vi "ORCAFusionfor3D250213.vi"(1 "V Offset":i32=1008 min=0 max=2004 step=4, 2 "Exposure":dbl=0.005 min=6.576470588235294e-05 max=10.000017235294118 step=1e-08, 3 "V Width":i32=300 min=4 max=1296 step=4) -> ()   [LabVIEW 2024]
uses:
  <vilib>/vision/driver/IMAQdx.llb/IMAQdx Acquisition Mode.ctl
  <vilib>/vision/driver/IMAQdx.llb/IMAQdx Buffer Number Mode.ctl
  Global variables/filepath global variable.vi
  Global variables/Global 1.vi
  Global variables/global for picoscope.vi
  <vilib>/Utility/file.llb/Write Delimited Spreadsheet (DBL).vi
  Global variables/Global for awg.vi
  <vilib>/Utility/file.llb/Read Delimited Spreadsheet (DBL).vi
  <vilib>/regexp/Match Regular Expression.xnode
  RIGOL DG4000 Series/RIGOL DG4000 Series.lvlib
  <vilib>/vision/driver/NI_Vision_Acquisition_Software.lvlib
  <resource>/objmgr/imaqdx.rc
panel:
  in  "use most recent 2":bool=TRUE
  in  "folder for imgcalib.txt":path=path "E:/20250409-103904beads-cropbulkcalib"
  in  "copy later":bool
  out "UDP wait":i32=236
  out "result":bool
  in  "force stop":bool
  out "time ofst":dbl=2434.2794585227757
  out "Image":u16[][](graph)
  in  "force 2":bool
  out "rec ready":bool
  in  "force":bool
  in  "master IP":string="192.168.11.3"
  out "Frame Count 2":i32=1726
  out "Frame Index":i32=1725
  out "error out 6":errorcluster
  out "error out 5":errorcluster
  in  "UDP send at monitor":bool
  in  "save BF video":bool
  out "error out 4":errorcluster
  in  "Stop (F)":bool
  out "BF save idx":i32=157
  out "Tot Img Trans":u32=158
  out "Lost Imgs":u32
  in  "error in 2":errorcluster caption="error in"
  out "buffers to read":i32=1
  in  "UDP send vol img":bool=TRUE
  in  "pico send port":u16=61558
  in  "pico receive port":u16=61559
  in  "cam receive port":u16=61551
  in  "cam send port":u16=61550
  in  "img send port":u16=61554
  in  "img receive port":u16=61556
  in  "img process IP":string="169.254.243.60"
  in  "slave IP":string="192.168.11.4"
  in  "ROI ratio [0-1]":dbl=0.40000000000000013 min=0.0 max=12.009207563363388 format="%_3g"
  in  "BF Gain":dbl=1.40920756336339 min=0.0 max=12.009207563363388
  in  "BF Exp Time [us]":dbl=25000.0 min=81.0 max=1000000.0
  in  "picoscope  IP":string="192.168.11.5"
  in  "control picoscope dependent enable":bool
  out "error out 3":errorcluster caption="config save"
  in  "avg":bool
  out "img projection on x":u32[](graph)=[46763, 46566, 47465, 47353, 48054, 49097, 50269, 51790, 53469, 55555, 57972, 59664, 62238, 64752, 68892, 72850, 78469, 84812, 92692, 100027, 109195, 119310, 130289, 140697, 155154, 168575, 186107, 203972, 224307, 243761, 265655, 286409, 306031, 324848, 342017, 357018, 368904, 379402, 387267, 388850, 395332, 391042, 392409, 389360, 387631, 382204, 372553, 361258, 353852, 348315, 349132, 352795, 362226, 378823, 399724, 419608, 438876, 459397, 481066, 502548, 524212, 537389, 551531, 567399, 572506, 575998, 579368, 577266, 572748, 565672, 554518, 543313, 531291, 514913, 503094, 495158, 488186, 477560, 468588, 467112, 458508, 452252, 445557, 436410, 425728, 418022, 407398, 396484, 384057, 369408, 354457, 334333, 315868, 295311, 272375, 251508, 229534, 206536, 185054, 162964, 142104, 125408, 111109, 98736, 88371, 80016, 75159, 71056, 66418, 63549, 62540, 60488, 59786, 59593, 58091, 58342, 57603, 57721, 57813, 58251, 57480, 56985, 56492, 55978, 55882, 55969, 55694, 54777, 55153, 54636, 54366, 54397, 54470, 54398, 53686, 53410, 52884, 53176, 51940, 51877, 51333, 51303, 50817, 50985, 50476, 51047, 50390, 52065, 53983, 54808, 55888, 57189, 58691, 60664, 61183, 62686, 64574, 67089, 71468, 75339, 80938, 88612, 96438, 106174, 117774, 131064, 143808, 162504, 179386, 199476, 221027, 241869, 264955, 289252, 314205, 339403, 360641, 381980, 400735, 413883, 425153, 437700, 437408, 441439, 438854, 433479, 429254, 421027, 412972, 405392, 396731, 386405, 373085, 362958, 361482, 367425, 375402, 388356, 414798, 445670, 475814, 507271, 539682, 567255, 593366, 615447, 634310, 648625, 657756, 659455, 652031, 647118, 635908, 619182, 600572, 575600, 548617, 521219, 489430, 463193, 440358, 414296, 395402, 379226, 362114, 347669, 336524, 321767, 311716, 298256, 290618, 283823, 275246, 264692, 257127, 245035, 235078, 222050, 207522, 192842, 179267, 165496, 150685, 136934, 122505, 112106, 99543, 90769, 83386, 77341, 73424, 69532, 66073, 63964, 61802, 60456, 60172, 58053, 58610, 57914, 57379, 56188, 56799, 56522, 56383, 56136, 56350, 55969, 55894, 55596, 55550, 54966, 54216, 55062, 54752, 54939, 54056, 54219, 54106, 53703, 52919, 52784, 52570, 51188, 51390, 51350, 50853, 51444, 51914, 53286, 54912, 56386, 57845, 59413, 61190, 61964, 62139, 63564, 65517, 66692, 68803, 72468, 75689, 81725, 88028, 96533, 106800, 119624, 134822, 150087, 169629, 188666, 213128, 237819, 265095, 290925, 321363, 352398, 380193, 407341, 429230, 449456, 468115, 478920, 483867, 493482, 494367, 495346, 491733, 479634, 470046, 458955, 444614, 433281, 422348, 410073, 402638, 392584, 389266, 392847, 405373, 422542, 450281, 484856, 524179, 564068, 600997, 635572, 667615, 693349, 710453, 723810, 733326, 733971, 727639, 712926, 695281, 673791, 644151, 611255, 574822, 533808, 489856, 452557, 413089, 378985, 344296, 316157, 288985, 267488, 246789, 230505, 217301, 205969, 197601, 191265, 186443, 180492, 173239, 168631, 161521, 154799, 147874, 139498, 133757, 122991, 117586, 109419, 101760, 94727, 87387, 81708, 76026, 72895, 69737, 65592, 64545, 61762, 61493, 60316, 58335, 58021, 56599, 56717, 56451, 56236, 55904, 55987, 56231, 55048, 55126, 55901, 55591, 54653, 54155, 54580, 54543, 54603, 53867, 54428, 54306, 54044, 53700, 53600, 53539, 53111, 53102, 52748, 52697, 53594, 55555, 57500, 58837, 61645, 64114, 65348, 65886, 67016, 67614, 67654, 69657, 72162, 75056, 78198, 82504, 88800, 96598, 106234, 117020, 131257, 145720, 164156, 182364, 203376, 229013, 257225, 289129, 316516, 351185, 379123, 410151, 437385, 462763, 481027, 499315, 510603, 518971, 520139, 522881, 518519, 516459, 512100, 498143, 485882, 475328, 460116, 450415, 437217, 426723, 420391, 413940, 412723, 419085, 432764, 456433, 485422, 524525, 565162, 610088, 648437, 686398, 718800, 747419, 766010, 777514, 777044, 778427, 763909, 751696, 725442, 695879, 665038, 625739, 585270, 539158, 490792, 441142, 394881, 350379, 311008, 274508, 243018, 216015, 191695, 172900, 158220, 144123, 135334, 129242, 125294, 121970, 118239, 115135, 113271, 108002, 105537, 103368, 98928, 96060, 92167, 88539, 85061, 81133, 76890, 73457, 69890, 68677, 66634, 64257, 61754, 60821, 59558, 58395, 58513, 56328, 56141, 55792, 55574, 55876, 55499, 55004, 55402, 55345, 54894, 54699, 55016, 55041, 54684, 54209, 54577, 54510, 55124, 53770, 53483, 53717, 52644, 53505, 53602, 53088, 52707, 53282, 55024, 57713, 60024, 62878, 66235, 68694, 71215, 72999, 75032, 75858, 78590, 79163, 82438, 84466, 88891, 93706, 101282, 108113, 117174, 128616, 140654, 156941, 173135, 189677, 209640, 233642, 255507, 284400, 314625, 343006, 373109, 405302, 430985, 454705, 479403, 499728, 509992, 522190, 534539, 537888, 540312, 541391, 536423, 533375, 527903, 521478, 511809, 497760, 490753, 481320, 470512, 463190, 455798, 455219, 457499, 463730, 483205, 501868, 534714, 570832, 612318, 653007, 688852, 726270, 755878, 773610, 786847, 793248, 788675, 778998, 762326, 741613, 710124, 680934, 645559, 600535, 559941, 510879, 462833, 411293, 361698, 316739, 276859, 238493, 206282, 177438, 155511, 136038, 121533, 111596, 102609, 98600, 93511, 91228, 90109, 87612, 86054, 84772, 83804, 83650, 81231, 79034, 78308, 76125, 74817, 73368, 71865, 69032, 66726, 66145, 64251, 63185, 62358, 60763, 59310, 58836, 58519, 57076, 57695, 56673, 56647, 56615, 56011, 56065, 55656, 55461, 55662, 55299, 55677, 55908, 55040, 55014, 55895, 55142, 55733, 54291, 54438, 53795, 54601, 55215, 55425, 56957, 59882, 62453, 65632, 68780, 72560, 75412, 79552, 81468, 85046, 88090, 91442, 94344, 97575, 102906, 109576, 119126, 127735, 135862, 149342, 163796, 178621, 197113, 214594, 234706, 252396, 273899, 294607, 316765, 343214, 368638, 393386, 420665, 442983, 464259, 480357, 492508, 500708, 510357, 516660, 524411, 530971, 535190, 536034, 537105, 535876, 532909, 533313, 526314, 519232, 511560, 501525, 495308, 483290, 479364, 479346, 478860, 483300, 492570, 510965, 535881, 562874, 596055, 632312, 662038, 696751, 717383, 742176, 749917, 755987, 746600, 739245, 721556, 703042, 678722, 646019, 613429, 576811, 534667, 494339, 446301, 397380, 352581, 306403, 267865, 228945, 197581, 171555, 148010, 128502, 114118, 103197, 94032, 87802, 82480, 81184, 79017, 77204, 76793, 75420, 74572, 75099, 73593, 73408, 71627, 71309, 70209, 70774, 68776, 67944, 66009, 64393, 64407, 61956, 62331, 60890, 60805, 59475, 58855, 57975, 58083, 56975, 56977, 57278, 56861, 56411, 57107, 56762, 56913, 56257, 55657, 56298, 55799, 55779, 55602, 56401, 54827, 54668, 54422, 55422, 56213, 58272, 60132, 62006, 66355, 68450, 72697, 76562, 79975, 84644, 88439, 94301, 98930, 105254, 111465, 118621, 126709, 135204, 146414, 159222, 173651, 191478, 209063, 229838, 250513, 272267, 291585, 314719, 332340, 352328, 371069, 388356, 408658, 424320, 444853, 460671, 475012, 485228, 494000, 494571, 499023, 498881, 501009, 508428, 513098, 522833, 531481, 533378, 538412, 541736, 542287, 540438, 537292, 533782, 527968, 518489, 511686, 501691, 492153, 489715, 486694, 488329, 492105, 504124, 520584, 539851, 562253, 586323, 615491, 635563, 651874, 659035, 662606, 657157, 647946, 637716, 618358, 600924, 574402, 546181, 516077, 486466, 446289, 412376, 372443, 330677, 292392, 255923, 221850, 192879, 167113, 145811, 127025, 113704, 102444, 94562, 87374, 83407, 77742, 77121, 74132, 73679, 72464, 72005, 71342, 70178, 70459, 69718, 69138, 68748, 68189, 67696, 66799, 65713, 64961, 64463, 63252, 62852, 61849, 60461, 59643, 59776, 58932, 57673, 57651, 57025, 56749, 57710, 58078, 56667, 57160, 56437, 56713, 55969, 55979, 55988, 55737, 55922, 56094, 55446, 56541, 57664, 59499, 61720, 63823, 66018, 69061, 72232, 75368, 79556, 82900, 87771, 93106, 100163, 109727, 119195, 129630, 140138, 153328, 168378, 184368, 202515, 226296, 249446, 274734, 300671, 326457, 349959, 375628, 399007, 417677, 438041, 451834, 467356, 477363, 487782, 497901, 507169, 513957, 516170, 513887, 514861, 513323, 507136, 502739, 499439, 502497, 509217, 519171, 531478, 539064, 548065, 553679, 558886, 560565, 555793, 553298, 548006, 535963, 526058, 509826, 501258, 489039, 480329, 467466, 459027, 455901, 457194, 466412, 472844, 481954, 500378, 515647, 527143, 528788, 532753, 529135, 521695, 511153, 497039, 478216, 461326, 438452, 420035, 397745, 368464, 341391, 311948, 280824, 253865, 222955, 195390, 170664, 149175, 132071, 118878, 108688, 99158, 91978, 87181, 83209, 79800, 76421, 74690, 72193, 71263, 70267, 70410, 69170, 69505, 69184, 69134, 68814, 67928, 67770, 66360, 66150, 66109, 64758, 63735, 63081, 61919, 61853, 61632, 60449, 60652, 60128, 59036, 59188, 59063, 58580, 57639, 58652, 58142, 58260, 58426, 58344, 57729, 57843, 57657, 58503, 60967, 62530, 64189, 67978, 69308, 72699, 75598, 76963, 78740, 82423, 86195, 90634, 96316, 104436, 113212, 123960, 135348, 151749, 167657, 187248, 208644, 234661, 261361, 289449, 318033, 347216, 382491, 411942, 443503, 470688, 494191, 513211, 532495, 546968, 559280, 563098, 568707, 574630, 576306, 573994, 574301, 572743, 565857, 556853, 550941, 541122, 530722, 527826, 530160, 537484, 545186, 560363, 573150, 583316, 583372, 584437, 577068, 574591, 566652, 556635, 544800, 530273, 510395, 490442, 472939, 452229, 428681, 407695, 388867, 377702, 370827, 370301, 368389, 371544, 379539, 384309, 387899, 387049, 383115, 373877, 365172, 358048, 345655, 332013, 320266, 301273, 287529, 269564, 252052, 234242, 214021, 193605, 174578, 156405, 139534, 124363, 113613, 106526, 99431, 93531, 88245, 84911, 81424, 78650, 76329, 74234, 72670, 71463, 69882, 70270, 70029, 69343, 68388, 68592, 68126, 68251, 67684, 67107, 66204, 66381, 65869, 65350, 64341, 63657, 62936, 63157, 62354, 62490, 62383, 61429, 61896, 60989, 60215, 60454, 59986, 59353, 60091, 60083, 60272, 61016, 61732, 63650, 66878, 69853, 72409, 76090, 77719, 81626, 83862, 84953, 88525, 91994, 95122, 100678, 106585, 115016, 123268, 134460, 148618, 166605, 184944, 207904, 229903, 260888, 290300, 322193, 358613, 392442, 424837, 465456, 501501, 532401, 561444, 584650, 607106, 623032, 635080, 645734, 653773, 656815, 658544, 656549, 654539, 647014, 646190, 638408, 627915, 619526, 606518, 599238, 589066, 588115, 587987, 596125, 605755, 616686, 623131, 626647, 621152, 609225, 597147, 582436, 566852, 555739, 537492, 514810, 491461, 466012, 439105, 410246, 379739, 348501, 319113, 299635, 283029, 271006, 259836, 257610, 255632, 255968, 256242, 254458, 250537, 245450, 240074, 234972, 227618, 218501, 211862, 202945, 193330, 183380, 173531, 162316, 151819, 141017, 130507, 119635, 110267, 103633, 97552, 92520, 88504, 84892, 82268, 79516, 78045, 75838, 74257, 73572, 71734, 70639, 70069, 70069, 68607, 68328, 68748, 69112, 67981, 67374, 67373, 66304, 66789, 65901, 66062, 64961, 63977, 65245, 64377, 63630, 63604, 63967, 62407, 63214, 62344, 61961, 61774, 61036, 62023, 62930, 65684, 66942, 69995, 76001, 78880, 83373, 86841, 89315, 93801, 94836, 97208, 101451, 106133, 111049, 118204, 124706, 134766, 147204, 161353, 175813, 195481, 216380, 238811, 261184, 292301, 320473, 353593, 390048, 424548, 461921, 498089, 530867, 564423, 595816, 626983, 652126, 671002, 688270, 701533, 713810, 722754, 726314, 729340, 732940, 733028, 731046, 726045, 715923, 704688, 696391, 687102, 683341, 670739, 663697, 661041, 660387, 662810, 669403, 670798, 664673, 656682, 637876, 617533, 589418, 567700, 551910, 532396, 509588, 482087, 454509, 425145, 391865, 358574, 321135, 285411, 254640, 230948, 209641, 195414, 181370, 174427, 167958, 165639, 164684, 160171, 157109, 155233, 153616, 149682, 146704, 142205, 137923, 134356, 129851, 124980, 120013, 114239, 108885, 103690, 99268, 94468, 90762, 86230, 83823, 81021, 78977, 77084, 75557, 74597, 73002, 72729, 71162, 69426, 70028, 69318, 67892, 68868, 67483, 66913, 67287, 67555, 66142, 66315, 67040, 65491, 65669, 65403, 65681, 65224, 65278, 64135, 64150, 63686, 64044, 63637, 63242, 62525, 61698, 62245, 61811, 63049, 64547, 67956, 70609, 75237, 81093, 85648, 93090, 97431, 101731, 106858, 110864, 117654, 122759, 129252, 137895, 145048, 155739, 170843, 185489, 204045, 223243, 243633, 268584, 292435, 317121, 342349, 369902, 399530, 429393, 462446, 496455, 529059, 558314, 587899, 616309, 644410, 666002, 690379, 708113, 731660, 751461, 765659, 782685, 791681, 799765, 805173, 808663, 812066, 807592, 797973, 788513, 775893, 762811, 751623, 741070, 729946, 720074, 717443, 716245, 709738, 702259, 693124, 681834, 662431, 636216, 604702, 574075, 544633, 520712, 497617, 477753, 447300, 416352, 386342, 350714, 316994, 279730, 245240, 215017, 186365, 165427, 149431, 134762, 124069, 117802, 113972, 111451, 108212, 106559, 106003, 104053, 102471, 101832, 99318, 97950, 95984, 94380, 92804, 90925, 87889, 86332, 84699, 81928, 79786, 78244, 76929, 74832, 73871, 71723, 71905, 70749, 69591, 69410, 68104, 67663, 67370, 66572, 65358, 65540, 65770, 65293, 65134, 64461, 64123, 64955, 63954, 63499, 64235, 62877, 63787, 62841, 63494, 62554, 61743, 62057, 61599, 60186, 60950, 60480, 60778, 60657, 62136, 63581, 65769, 69642, 74391, 79857, 85246, 92397, 98998, 107390, 116571, 124545, 131994, 142229, 153291, 163548, 177881, 191992, 207585, 230523, 250293, 273919, 300201, 327896, 357657, 380818, 409210, 434937, 462041, 486284, 512740, 539203, 565531, 588857, 619273, 636650, 657509, 678060, 694261, 715038, 735168, 759656, 775484, 795112, 815744, 839395, 851805, 862003, 870832, 874827, 874824, 869134, 856216, 841567, 821890, 802659, 784915, 768650, 751584, 741555, 731571, 716175, 702050, 688414, 676278, 651137, 627903, 598903, 562873, 530382, 502630, 474887, 452077, 428903, 404965, 378811, 347369, 316651, 285902, 253523, 219876, 191077, 162607, 144229, 127086, 114637, 105398, 97788, 93173, 90056, 87082, 84545, 83619, 83178, 82178, 80760, 79681, 80028, 78757, 77506, 77230, 77014, 76447, 75667, 74473, 74658, 72432, 72148, 71246, 69164, 69417, 68323, 67018, 66728, 65535, 65955, 64540, 64052, 64783, 63809, 63934, 62562, 63125, 63382, 63195, 62089, 62263, 62538, 61898, 62003, 61987, 61715, 60810, 60764, 60289, 59903, 60112, 59165, 58832, 59077, 60239, 60941, 61907, 63578, 65479, 68861, 72721, 78549, 85103, 92676, 100742, 110143, 122825, 137696, 151108, 165849, 181928, 200582, 219123, 240759, 268390, 293942, 322516, 350804, 380186, 415968, 450931, 481132, 512024, 543238, 572639, 595963, 623884, 641402, 667756, 685579, 704673, 719769, 734097, 746735, 756245, 763244, 776213, 785879, 797241, 809994, 830952, 853748, 884065, 898879, 915910, 924958, 929875, 921709, 913768, 902456, 880502, 852432, 821412, 791564, 758247, 733464, 713488, 694840, 679243, 660419, 640481, 619488, 593945, 573547, 543351, 514023, 481765, 451702, 421292, 397609, 376451, 358299, 337797, 314412, 292551, 265775, 242066, 213026, 187817, 163852, 144755, 127914, 114425, 102441, 96208, 90535, 85740, 82498, 79334, 77852, 76006, 75789, 74410, 75163, 73839, 73611, 74269, 72906, 73256, 72890, 71503, 71628, 71277, 71731, 70354, 69625, 69495, 68541, 68131, 66889, 66153, 65214, 64926, 65725, 64831, 64657, 64172, 63755, 63769, 62687, 63541, 63148, 62709, 63217, 62308, 62666, 62670, 62457, 61548, 61571, 61103, 61423, 60534, 59216, 60958, 60785, 61214, 61294, 63337, 63371, 65573, 67443, 69870, 74322, 78052, 84778, 92348, 102626, 112453, 127034, 144489, 166031, 186787, 212098, 238712, 272078, 303589, 336952, 373906, 413511, 449802, 488112, 529905, 572761, 612162, 649537, 684337, 717353, 747525, 780325, 799854, 821516, 842427, 860436, 870764, 876368, 887719, 886533, 886338, 884878, 882939, 878119, 876774, 883135, 887243, 902900, 928355, 950250, 958519, 964094, 967841, 958992, 935840, 917902, 884201, 852477, 806465, 763670, 720665, 681044, 649302, 622608, 599953, 576659, 551065, 526067, 503866, 474630, 449745, 423022, 396999, 370839, 344772, 323190, 302128, 288776, 273658, 258814, 242313, 221669, 204526, 184526, 166382, 151290, 133572, 120289, 109493, 102207, 94856, 91292, 85823, 82481, 81064, 77533, 75875, 75553, 76188, 74126, 74914, 74264, 72800, 72663, 72818, 71612, 73391, 70575, 70713, 70828, 70331, 69837, 69740, 69456, 69369, 69092, 68393, 68244, 65885, 65892, 66170, 65288, 65606, 64420, 64465, 64831, 64243, 63648, 63970, 63360, 63355, 64023, 62883, 62986, 61553, 61221, 61975, 61749, 62484, 62149, 62848, 63036, 63655, 64647, 65540, 66994, 69767, 70452, 73899, 76465, 81806, 86263, 94014, 102961, 115672, 132973, 151256, 174915, 202830, 235405, 270932, 309650, 350970, 402340, 447192, 496732, 541670, 594440, 647322, 690986, 742780, 788664, 829420, 872703, 911922, 945992, 967093, 995894, 1023769, 1044035, 1055736, 1065514, 1067810, 1067918, 1062822, 1056107, 1040368, 1023694, 1004512, 987379, 966399, 958464, 953263, 962909, 973305, 982364, 977187, 967864, 949521, 921940, 892684, 857498, 815282, 763596, 711178, 658337, 607590, 563858, 527965, 500003, 469418, 446141, 419065, 394736, 371463, 347798, 325460, 304621, 286410, 262655, 246715, 231281, 218527, 207951, 196175, 186747, 175289, 162510, 152076, 138768, 127521, 118057, 109188, 102916, 96430, 92342, 88799, 85983, 83518, 81444, 80225, 77409, 76879, 74841, 74356, 74110, 73313, 73319, 72944, 72192, 71987, 71450, 71381, 70868, 69768, 70381, 71173, 69571, 69147, 69153, 68938, 69572, 68696, 66881, 66746, 66779, 67580, 66299, 66488, 65587, 65330, 64789, 65169, 63458, 63127, 64178, 63283, 62548, 61478, 60982, 60950, 60289, 60191, 60949, 60917, 59272, 60064, 59752, 59923, 60254, 60326, 59469, 58715, 59647, 59200, 58036, 58655, 57850, 58271, 57778, 56639, 56055, 56910, 57189, 55912, 56106, 56456, 57093, 56121, 57182, 56239, 55974, 56403, 56361, 55629, 57655, 55400, 56492, 55490, 56104, 56031, 55803, 56218, 55837, 55851]
  out "x-y":i32=1726
  in  "calib":bool
  in  "page":i32
  in  "calib/monitor":bool
  in  "max adjust":dbl=1.0 format="%_2g"
  out "frame's init pos in x":dbl[][](array[numeric])=[[0.0, 0.411157223986379], [140.8042176643056, 140.13608717532782], [280.2664638336562, 281.07735724762904], [420.37970894098385, 420.73947151197183], [560.413006810315, 560.8241640343012], [700.4177520946471, 700.3663574416489], [841.3247590649489, 840.9649964939609], [981.1581888392866, 980.7184790303013], [1120.4405537231426, 1120.9002503416273], [1261.6530733529344, 1261.807257311929], [1401.606423984268, 1401.1952667602816], [1541.9480897715885, 1542.2564576895784], [1682.0013744504195, 1682.700912782896], [1822.705658067228, 1822.9626313322192], [1963.5013099560329, 1963.2471919495415], [2103.2576477508737, 2103.463226362867]]
  out "stop acq":bool
  out "cropcalib ch2 2":dbl[][][](array[numeric])=[[[0.8701974985351326, 12.622808311820734, 0.34821884375588075, -0.03186060376885538], [0.7855164449626466, 12.248049490220744, -1.7933514926448941, -0.02615765607541458], [0.8790915308550922, 12.649388072757741, -1.7193702597053502, -0.03530778831987937], [0.8898204410615707, 12.542700034696967, -1.2340309712985338, -0.0439179338550789], [0.8871233001173581, 12.211143396475, -0.7011267129566395, -0.04065012404196286], [0.8976455855239693, 12.395744078277922, 0.44657632622208226, -0.035478990396647044], [0.6373130758818424, 10.721989467950603, -1.4081455713558404, -0.03444993212203115], [1.0111876965038278, 13.101523969448772, -1.3515523786356038, -0.006328878978959408]], [[0.3516942877029585, 4.921154461560632, -1.4770116333666226, -0.044838979986691584], [0.4586265170701861, 6.290835239491175, -0.5978805404070313, -0.03058477703735147], [0.48928552986839696, 6.246479501151768, -0.8501187541827993, -0.038934055058172115], [0.4704781032593286, 6.085031903419253, -1.2048861241864888, -0.027245570005914273], [0.4829021826517912, 5.720772505452486, -0.31646170698518505, -0.03774629427187434], [0.47432244943347757, 5.744490489126907, 0.3764850609397732, -0.026645671939902214], [0.35735176873885377, 5.155667320753812, -0.6110375964837094, -0.043001090221026814], [0.47169885007454965, 5.719049879710236, -1.214570394374455, -0.0357302420415391]], [[0.42431543103473984, 3.311153310021567, 0.3735087392794577, -0.026078458785932162], [0.4185393774710084, 3.510033946713933, -0.6974826786495143, -0.023717547547826606], [0.40107970241405455, 3.155388779364144, -1.4495184075110343, -0.0272149970173807], [0.4038785451829636, 2.894250692768182, -0.6626971578268964, -0.0325936670560735], [0.43463410117317575, 2.814665468074131, -0.07031969386775042, -0.02770361073912457], [0.45431959379871734, 3.3728460691517603, 0.04004989854315301, -0.02424459784876358], [0.4505805120561091, 3.337447688751297, -1.2625490394650989, -0.026776561893721327], [0.4251020680903856, 3.127743751549204, -0.6429568474166446, -0.02863037070461889]], [[0.3552757546386318, 1.3397492427317914, -0.3215132994421062, -0.025808768004406273], [0.36295246493286104, 2.0006437609736487, -1.3336461209741413, -0.017833549159850304], [0.35855770640942686, 1.8571434623079024, -1.4041148558396288, -0.020755845044606074], [0.4114652020285343, 2.0139473340600365, -0.1937946219538823, -0.02382442826394008], [0.3499301521182933, 1.3389264069092857, -0.21029767748849823, -0.022723031905148013], [0.38059424489364246, 1.5220229333510222, -0.1302571590494475, -0.016263248981750543], [0.4207868671061959, 1.9890909149992932, -0.11465078250135777, -0.019859715040226194], [0.4148040618017305, 1.6458278151709658, -0.41822866513797036, -0.02596361679279958]], [[0.2938047023063933, 0.15848081496267857, 0.21377935785301977, -0.017044009015294515], [0.3578200533394036, 1.440800298674786, -0.25425224089524223, -0.013068948485870282], [0.35091888359219314, 1.346093085991901, 0.03700652414677099, -0.018437088761087322], [0.2615412035983308, 0.2553357946660699, 0.06563804987560529, -0.013729022790036183], [0.27744688808915585, 0.16285376720024541, 0.3969513138143117, -0.024167766761933995], [0.2410317694018692, 0.01719906807802845, 0.31887980936003024, -0.013899480418623898], [0.32670519203836695, 0.7070294256236573, 0.06889024493523768, -0.013849213382843669], [0.26929735820100886, 0.21585137293623718, 0.16764603161195335, -0.017509725152931335]], [[0.23964527052154094, 1.405161828042007, 0.7263938040790185, -0.013558480972783012], [0.23329678829132916, 1.9842641685831914, -0.43751729409466744, -0.009372812399959492], [0.29609136804454006, 2.2197331529484727, -0.3606187984687732, -0.014591349298057148], [0.18364046988106897, 1.0318842702071733, -0.21467102230538426, -0.006974976860324521], [0.237430149883509, 1.1354461619807799, 1.253426813991111, -0.010764567951424628], [0.21428788494745543, 1.2084708667209956, 0.6454519731653344, -0.014856742787382637], [0.19128550557336332, 0.9914202026492045, -0.012966520111932736, -0.01039845002841516], [0.18478085458589122, 0.6855671795600868, -0.05129936188141995, -0.014242565681526993]], [[0.15123693469828958, 1.163110201653609, 0.8745656657567553, -0.006604690732614436], [0.1617626592665295, 1.8451285513720417, -0.22859918528260925, -0.006219911053321165], [0.16565366259007014, 1.6280136877205398, -0.10883101331753334, -0.00964042687757254], [0.10928971110762957, 0.749493310399407, 0.003138228221609993, -0.008573046658971014], [0.02253022817352303, 0.07522041477715277, 0.8174746482416958, -0.007898334309960686], [0.003821773667235064, 0.19087983139285825, 1.2250839805129892, -0.006940107606339307], [0.17999809793891175, 1.4975328046377405, -0.11799490261557272, -0.0031203973369017474], [0.12067298238529153, 0.8183571646791823, 0.21700018598403456, -0.003330307143816533]], [[-0.0005213232213452705, 0.11664433274256322, -0.14703000948528538, 0.0022223370156425545], [-0.004751436308695322, 0.44945437865127735, 0.4407582496415892, 0.0009313311130397984], [-0.04601125513680242, 0.12232865474884935, -0.5555144671157969, -0.008711753743847687], [0.0, 0.0, 0.0, 0.0], [-0.0006907142392795103, 0.0644444433024974, -0.0722068891602118, -0.0030870140283082302], [0.001947573415548731, 0.009430552383996885, 0.376950878453279, 0.004011208280281968], [0.00601799297429685, -0.171200104000229, 0.4028188227208616, -0.0006892635684963884], [-0.0035595026932949752, -0.1639845558444737, 0.20081933970234833, 0.0007759675622934727]], [[-0.0445905899107714, 0.3878308646235794, 0.2999945087607148, 0.0006132606194773083], [-0.0233479900245816, 0.805464715742334, 0.002260800741456181, 0.0007923205997293554], [-0.027075628767392633, 0.21947910469952261, -0.6085871209249598, -0.00044238879126859074], [-0.14801341061316545, -0.9604402676156238, 0.04927742722480564, -0.010081622437758307], [-0.1351946090418747, -1.4037614517100776, 0.19096669008196027, -0.0005919410201843423], [-0.025443865945330033, 0.16995044160417527, -0.1562744263326309, -0.00198507171588911], [-0.017148669006657007, 0.20096477942386526, -0.0948436802257652, -0.0037168132796431656], [-0.045635057561963205, -0.07042763819321216, 0.178354420444418, -0.001384743167300897]], [[-0.14847892629844361, -2.1190919588657353, -0.39668969526474496, -0.003525009441780651], [-0.15170487526883455, -1.517780253977753, 0.40100295859357254, -0.003671659512345847], [-0.15582312230276163, -1.749691739278918, 0.4041461560506011, -0.006519857435921785], [-0.1490680046293541, -2.141748665352092, 0.4764301961883949, -0.0037233647798519207], [-0.19546209831376074, -3.094433551917896, 0.10995617619126552, -0.0013108345240767923], [-0.1663997352333837, -2.5234347104959314, 0.016952984209117655, -0.001558016324829012], [-0.16864610100772026, -2.2519891134627716, 0.009421852652772325, -0.0015948467476679916], [-0.17038719997008178, -2.6042474433647995, 0.09965476021822894, -0.0009880362442417799]], [[-0.1917409778980073, -3.892103482576627, 0.011307393107903144, -0.000973113351354111], [-0.23155366010446854, -3.73698000173536, -0.32159229488976254, 0.0043611241773148105], [-0.2149861492875637, -3.826512088064914, 0.35988121969000053, -0.003276087734406148], [-0.1850914206691932, -3.9073215173591516, -0.2976902305965188, 0.0018181088617474789], [-0.2166956185114457, -4.759035950022652, -0.39731132566536975, -0.0018975172421048176], [-0.18453416290159624, -4.081079332925176, 0.06634914312032889, 0.007699054345041634], [-0.18380968001623293, -3.94398458212836, 0.05540268327058757, 0.0077636042799711326], [-0.17894442370330435, -4.023445572474, 0.174749370962602, 0.005127314289389062]], [[-0.2071791595959074, -5.602941921550978, 0.5697348661401064, -0.004793728154630928], [-0.293851025233213, -6.076200837157158, 0.36633789088880986, -0.014666619442646871], [-0.3125311419595355, -6.474337848680638, -0.46570696369851816, -0.012047430951543585], [-0.2759968219061918, -6.572782260152643, 0.26886806477602143, -0.012852068603061987], [-0.2936587113768818, -6.974886539171132, 0.8883198818115932, -0.012730943822099026], [-0.23093202328582216, -6.1827075386667865, 0.9316427529555751, -0.012210883924464684], [-0.28464868233601415, -6.72909589800129, -0.19611855518100219, -0.00903527061959048], [-0.2625995405221107, -6.8102546031636955, 0.02108551835502591, -0.015084825328907772]], [[-0.017109063375111363, -6.305395147464962, 0.8493065447613946, -0.0027315707279580337], [-0.025183233654072573, -5.719115295608953, 0.25604355824758657, -0.0008328457993723413], [-0.011810426477860672, -5.756876322861796, 0.037077228631617845, -0.00508825489568598], [-0.021815470429823007, -6.764253867141102, 0.7528849605016921, -0.001718709211005901], [-0.017242461928480585, -6.867507311676377, 1.2998216029802259, -0.003178406222625727], [-0.1367473207454842, -7.368894585862941, 1.2187395147519533, 0.0011206638129489343], [-0.13939835532615258, -7.51839746503113, -0.16250224198741448, -0.008004712668605848], [-0.019153970264270632, -7.0125243850261025, 1.3284409701928372, -0.004219811523833364]], [[0.019682306949207716, -8.419884602382986, 0.6732033220764355, 0.0015869408442581077], [0.1342676842136754, -7.524039725140825, -0.37431134795767795, 0.003773576453475305], [0.1314848286265471, -7.858634951598969, 0.4067984956167212, -0.00041680645119449424], [-0.0023769326802557484, -9.435599598027125, 0.04226250370073082, -0.0045766590234569745], [0.11415934582312011, -8.967065961888935, 1.1616912507982886, 0.0017424276137151474], [0.006886096932619226, -9.124538610282109, 1.3445567104771639, 0.0021914730965736707], [0.0011853546556687636, -9.42889296285466, -0.09425767127590956, 0.004899855600506488], [-0.0031300437858024876, -9.620240941440606, -0.02985151339072315, -0.0035285519984824773]], [[0.19158100537043612, -9.973878447787747, -0.006863624293562527, -0.005091277194434075], [0.26447987114487426, -8.724786342424533, -0.07774075287962218, -0.004724860309786319], [0.1996364939410272, -9.360313632123415, -0.8082526536375445, -0.0056144966941685925], [0.2084764480893021, -10.169127800537426, -0.03308889327708536, -0.002301697763028448], [0.2372275579557133, -10.250819861501277, -0.056431256502948675, -0.0038013832607461037], [0.1922509036033489, -10.281680271187199, -0.16106822688380604, -0.0038161217587472586], [0.20343667754654882, -10.455658775951685, 0.04638001027351282, 0.0004225148653823805], [0.20924605109911876, -10.645286383709237, -0.2560681558188696, -0.009009170704748135]], [[0.8324350254386008, -7.5738976594623715, 0.014329030602573734, 0.006901506367214101], [0.8319769111866963, -7.325862948770705, -0.8312681835893114, 0.010517963078141769], [0.8353323200023774, -7.535011597070012, -1.3023747225436964, 0.0021814193999445996], [0.8316841554801186, -8.243511372338293, 0.0007712661209171201, 0.004297280031524099], [0.8325965528064283, -8.383550047857502, 0.07709444913444323, 0.0065460209544277795], [0.8801192911648763, -7.647708169014859, 0.16465071042293827, 0.004311475678621823], [0.9081305422228638, -7.550188011285636, 0.06288874368262504, 0.007952893331817507], [0.7179312827937098, -9.41628946575151, -0.14327709681944711, 0.0048404562595646735]]]
  in  "xy cut pos correct":dbl[][](array[numeric])=[[0.0, 0.0], [0.0, 0.0], [0.0, 0.0], [0.0, 0.0], [0.0, 0.0], [0.0, 0.0], [0.0, 0.0], [0.0, 0.0], [0.0, 0.0], [0.0, 0.0], [0.0, 0.0], [0.0, 0.0], [0.0, 0.0], [0.0, 0.0], [0.0, 0.0], [0.0, 0.0]]
  in  "cropcalib":path
  out "cropcalib":bool
  out "cropcalib ch1":dbl[][][](array[numeric])=[[[0.6932908559775823, 10.949810302135091, -2.4603685163177973, 0.07408273808786627], [0.016724289546730317, 6.728542937861516, -2.462801283818857, 0.06332729673597925], [0.9420961881441432, 12.472737571945348, -2.233583333518718, 0.0859905806444957], [0.8383089445100997, 11.707715807570054, -1.804451383440766, 0.07045945607246644], [1.0291484339413137, 12.445681344070865, -0.6175311500159801, 0.09873969807341883], [1.0846966396391728, 12.782884092082329, -1.4634208669301922, 0.0487163594468301], [0.842368540007493, 11.514421287056944, -2.238875549709322, 0.10079951259488677], [0.8062337603642507, 11.51605615548647, -2.311199370765047, 0.07570748649093449]], [[0.3418032121533898, 4.058253793563666, -1.463672632158616, 0.026412744534673453], [0.6094536159908467, 6.415336272579176, -2.2778661837714314, 0.04883602397324521], [0.3806338804663636, 4.899895285815402, -2.4233572060241437, 0.03805641890968792], [0.4860425458136212, 5.427211752946015, -1.9354125604420873, 0.06725611435968222], [0.550389528196239, 5.453186708216613, -0.7788956205646569, 0.07672970838709745], [0.5329410882079375, 5.689715152526323, -0.599550933028322, 0.06689487324608506], [0.4643479172147251, 5.1647085596871865, -2.4162013638300635, 0.0624696412548246], [0.3533663573164656, 4.364971139391912, -1.4268063404280085, 0.06068943315424949]], [[0.3869164423326841, 1.8844659507207409, -0.9639119970413876, 0.02942923937537905], [0.43724901016747486, 2.5856207741269017, -1.1906004316986105, 0.03958302177432739], [0.40004426859399467, 2.0647357875345764, -2.0659149584619136, 0.03859299919181695], [0.46541001821760375, 2.1384388307742537, -1.4073482666086865, 0.04488308910822736], [0.3576203372644601, 1.153764601451798, -0.5928754358056261, 0.047609175965134365], [0.46638078955843176, 2.2697143184804762, -1.1918576177380253, 0.04504323614046597], [0.45157388119125713, 2.267257282862441, -1.3357251932395797, 0.04652597808158525], [0.43096176882428744, 2.0474492939035187, -1.071741932033162, 0.03724331012975539]], [[0.3838172580406991, 0.8028318952138043, 0.0588908617678892, 0.01444616428356257], [0.343461889766013, 1.1475915709209357, -0.6588547703102442, 0.015803554088355664], [0.3763987828679226, 1.1712063846579135, -0.6769074189655186, 0.024228007246127607], [0.3530856408935865, 0.8342611264026852, -1.4387190173979956, 0.010483194207102042], [0.4021625754778446, 0.9182306660798015, 0.06562652758278997, 0.01641982954537009], [0.3818050284782834, 0.9880724260083877, -0.13785602994787427, 0.02379001313820476], [0.35429696926293436, 0.6813083173793655, -0.6963112945835426, 0.016435724288551987], [0.3702521545824984, 0.8260322313286419, 0.06580476931422152, 0.01974239849632977]], [[0.3251295288854647, 0.08162951243296128, 0.0790008379733502, 0.008351533342438426], [0.3184116597115484, 0.6389146793528593, 0.02157800461323737, 0.010772431460404613], [0.33430272672049394, 0.8503104333529756, -0.5502477872619949, 0.005656325288736127], [0.3530349094651437, 0.5861130647258975, 0.25078513210674735, 0.013829557001144077], [0.3436380458170871, 0.2904325635668302, 0.26360742518440283, 0.00921377547553684], [0.31019734685578226, 0.25509658388618417, 0.2223906110711863, 0.013622110979762314], [0.30999850825872943, 0.11132718524549548, -0.0559931894237939, 0.009396616486070819], [0.35443287240480026, 0.5933107991178024, 0.014970176567496721, 0.01221759834679446]], [[0.21893324230395655, 0.4307017894054972, 0.9271930992492656, 1.1255617397010035e-05], [0.2381242177135166, 1.0373535983687603, -0.3285865261031004, 0.0024299717182164624], [0.2763249098501036, 1.2484979145043877, 0.0863076193103606, -0.004360256711920413], [0.2206532806299601, 0.49633421203690287, 0.26579829054475673, -0.0006510305946989241], [0.19202411545757092, -0.13373575836068607, 0.02973627729876939, 0.002856848781370643], [0.20793334369039884, 0.09013464766791571, 0.2932865458848708, -0.0008086166081327471], [0.2609457513377248, 0.8348592892836849, 0.05299755985931702, 0.002732493111870288], [0.21198256459214565, -0.06622318971780507, 0.31127732837081545, 0.0007558065355999486]], [[0.02198049102168039, -0.14043026792898658, 1.374683430256279, -0.0036775227652195317], [0.006474785373919158, 0.15763577028697073, 0.025186590222700252, -0.0035895101522373323], [0.028928847220157643, 0.1086175139746498, 0.21177571019966546, -0.008729181949374755], [0.02109753103084888, -0.19241276648380545, 0.3666338592909282, -0.005771106872513677], [0.15543148795513193, 0.3610660861634742, 0.29093224244151983, -0.004157459970243882], [-0.000905727760535128, -0.10595129763436201, 0.27146654607673215, -0.0018575991305460444], [0.029016101284026166, -0.015888786606554323, -0.27005209657751583, -0.0009923606568790384], [0.021806215519704557, -0.1901261518105019, -4.509431596944725e-05, -0.0005050493970899936]], [[0.0051345937020069905, 0.1417958307994553, 0.11676223631539559, -0.001299280131670754], [0.003225405788820734, 0.5269979078326332, 0.15848080101589623, -0.005358065059918588], [0.01934334196570406, 0.3237617201127715, -0.175512477075023, -0.008459576903803475], [0.0, 0.0, 0.0, 0.0], [0.0022520487829248937, 0.1175068279333371, -0.3166806090286468, -0.006191375307516113], [0.0013151237976528239, -0.008535567339032416, -0.03556758643251224, -0.00012224007809625645], [-0.0034632651085103588, -0.2379851872116246, 0.4421064863210053, -0.005119973842237064], [0.01735488906941737, 0.007045086674791981, 0.09396637975998104, -0.003692211833540197]], [[-0.00010446054088301322, -0.18412356621397336, 0.41847308291107604, -0.008062397556328081], [-0.02300375817862533, -0.1118611173318975, 0.07671956192092533, -0.0059291943100168755], [-0.14752224338514275, -1.0222007519452783, 0.2960234309125709, -0.014386504725464237], [0.0034628278633417288, -0.34748121965799283, 0.27765853166130383, -0.013969112406284075], [-0.02551561505677409, -0.9341788503148312, 0.43997020554181887, -0.005556247344849434], [0.004048662007891117, -0.5692057447960979, -0.3971785327787668, -0.008977161410123417], [-0.07654940849790373, -0.9993731536492388, 0.37108473970379025, -0.013252252630013808], [-0.0055996778073565704, -0.6367977287734977, 0.4754587729738224, -0.009221465832238776]], [[-0.1418289244268497, -2.100828486313175, 0.1861904410089224, -0.017382956048777654], [-0.16992495348915698, -1.8274737296432406, 0.37042676552155984, -0.01637747522920484], [-0.17359675003932404, -1.974027313470481, -0.09178912509532614, -0.019832136461419708], [-0.12823692706307072, -2.1131743543163686, 0.39274574272543966, -0.020351859532969533], [-0.19797296352124533, -3.1206911804808426, -0.1435834558987767, -0.01659105732153679], [-0.20703741665898548, -2.893071312337848, 0.24388835808283565, -0.016102013318630072], [-0.033342690091984886, -1.496642532470326, 0.2891533008881042, -0.016347132935728616], [-0.11664903151594058, -2.2609875954496896, -0.4489814971826575, -0.01238293967294482]], [[-0.17534936811406382, -3.5136373648387567, 1.405523915677739, -0.024315231666195744], [-0.27493680225147943, -3.855974606871774, 0.35860056551148195, -0.02262388962743494], [-0.26190503548651556, -3.9631679301817906, 0.03336912243432735, -0.02814753332121247], [-0.1715867617685295, -3.6606468796107645, -0.4326034902949836, -0.009420120493471325], [-0.21331674497614084, -4.414287355708269, 0.8078932443062334, -0.019710489365945806], [-0.17982890727352507, -3.870559230926661, 0.8333789506155658, -0.020853514034276092], [-0.21996253232475796, -4.071356644886755, -0.19323564005647492, -0.02042596094833741], [-0.2035274261803407, -4.024820360860676, -0.10040296146174832, -0.02025809671502492]], [[-0.19676096357515788, -5.6716261896370455, 1.2538944632770406, -0.013267898567108485], [-0.20820796694322408, -5.590581172566877, 0.07242487176497986, -0.017019178578354957], [-0.23883760276332028, -6.076309700057891, 0.36914031013932996, -0.01544852619696964], [-0.1712303115237802, -5.690330488663776, 1.3118017771920882, -0.014743141732072768], [-0.21724137455845993, -6.338386734172362, 1.4780514405644967, -0.009724660532719842], [-0.16200648760963837, -5.762567817298242, 1.296335087630152, -0.01448488504045957], [-0.17383744446780913, -5.962786456204089, 0.7905580990129195, -0.009532711692076472], [-0.18224404603932998, -6.2000414424742365, 0.6887266289444529, -0.013601135108830906]], [[0.0013810792592013111, -6.197636972818618, 1.134475998910681, 0.06610347544209882], [-0.024143960252901737, -5.541498434717905, 0.6401075021764084, 0.06152559675677685], [-0.016335379031749815, -5.74982396726343, 0.17487268627387134, 0.05502998345567061], [-0.013849883235718148, -6.676229120352952, 1.3938437778467188, 0.06519564935275048], [-0.0006081400458059067, -6.709986155055729, 0.6416087760221056, 0.061425987304154356], [-0.14048656665500311, -7.30431082452389, 1.4441723096044505, 0.06539368629484452], [-0.09289241809423823, -7.201344724614182, 0.7405342969721602, 0.058037331627497586], [-0.013374881754029993, -7.012123585009522, 1.4185576139696165, 0.06425242473709128]], [[0.023828012980635548, -8.36273804175405, 0.8700140027744819, 0.2504094103941477], [0.1718253266301483, -6.943820572969749, 1.0824764128262592, 0.2332591085511838], [0.01500555618632084, -8.216737570365769, -0.1853635411371917, 0.2319052288032102], [0.020838954687245025, -9.029385123936752, 0.7346737266296544, 0.2274016223334501], [0.02824334053381549, -9.016036610808833, 1.0689532197527138, 0.23879170919198756], [0.11614361764338521, -8.042367916979941, 1.0540646011885904, 0.24018508832157548], [0.09274447960799986, -8.346772040027158, 0.912405906880001, 0.2497610644165143], [0.027219934829350034, -9.21449836460651, 0.6942519365012636, 0.23420249830563614]], [[0.4398984104611475, -7.950109888937487, 1.054541597316132, 0.4880491338769315], [0.4216658853169885, -7.486392930341779, 0.10919025723416158, 0.4851737849040064], [0.42192794062291394, -7.557335489018286, 0.1673158213306376, 0.47058265482703643], [0.44176005097680926, -8.148910837209007, 0.7987755229585237, 0.488474379048908], [0.405091788484518, -8.745554290197076, 1.1853789641980823, 0.48986502641939567], [0.3830572933143733, -8.484408380575875, 0.8555638763353651, 0.48912255761769263], [0.46322681455679393, -8.172649294320621, 1.2810836612962349, 0.496170340637091], [0.43964673545099714, -8.649576408260469, 0.6760470541669921, 0.4893302941674038]], [[1.0392599697907308, -6.435434121825245, 0.8696672987885002, 0.8274169673637829], [1.028614244674245, -6.5479644747285, 0.026315197400719276, 0.8339980063409057], [1.0313347040947445, -6.5136442834641475, -0.41002027099231003, 0.8141893556290383], [1.0055769666010141, -7.330480953954483, 0.7575147465354397, 0.8235395332184119], [1.302285769730466, -5.414687509396991, 0.895742660453535, 0.8336519226593232], [0.952727767848623, -7.217098526677311, 1.1427105333174121, 0.8339301485564363], [0.9851831581678892, -7.344320410840666, 0.08727111073827454, 0.8078336835332718], [0.9242892120571478, -8.434270883821462, 1.1802002020091944, 0.8351531236339481]]]
  out "cropcalib ch2":dbl[][][](array[numeric])=[[[0.8701974985351326, 12.622808311820734, 0.34821884375588075, -0.03186060376885538], [0.7855164449626466, 12.248049490220744, -1.7933514926448941, -0.02615765607541458], [0.8790915308550922, 12.649388072757741, -1.7193702597053502, -0.03530778831987937], [0.8898204410615707, 12.542700034696967, -1.2340309712985338, -0.0439179338550789], [0.8871233001173581, 12.211143396475, -0.7011267129566395, -0.04065012404196286], [0.8976455855239693, 12.395744078277922, 0.44657632622208226, -0.035478990396647044], [0.6373130758818424, 10.721989467950603, -1.4081455713558404, -0.03444993212203115], [1.0111876965038278, 13.101523969448772, -1.3515523786356038, -0.006328878978959408]], [[0.3516942877029585, 4.921154461560632, -1.4770116333666226, -0.044838979986691584], [0.4586265170701861, 6.290835239491175, -0.5978805404070313, -0.03058477703735147], [0.48928552986839696, 6.246479501151768, -0.8501187541827993, -0.038934055058172115], [0.4704781032593286, 6.085031903419253, -1.2048861241864888, -0.027245570005914273], [0.4829021826517912, 5.720772505452486, -0.31646170698518505, -0.03774629427187434], [0.47432244943347757, 5.744490489126907, 0.3764850609397732, -0.026645671939902214], [0.35735176873885377, 5.155667320753812, -0.6110375964837094, -0.043001090221026814], [0.47169885007454965, 5.719049879710236, -1.214570394374455, -0.0357302420415391]], [[0.42431543103473984, 3.311153310021567, 0.3735087392794577, -0.026078458785932162], [0.4185393774710084, 3.510033946713933, -0.6974826786495143, -0.023717547547826606], [0.40107970241405455, 3.155388779364144, -1.4495184075110343, -0.0272149970173807], [0.4038785451829636, 2.894250692768182, -0.6626971578268964, -0.0325936670560735], [0.43463410117317575, 2.814665468074131, -0.07031969386775042, -0.02770361073912457], [0.45431959379871734, 3.3728460691517603, 0.04004989854315301, -0.02424459784876358], [0.4505805120561091, 3.337447688751297, -1.2625490394650989, -0.026776561893721327], [0.4251020680903856, 3.127743751549204, -0.6429568474166446, -0.02863037070461889]], [[0.3552757546386318, 1.3397492427317914, -0.3215132994421062, -0.025808768004406273], [0.36295246493286104, 2.0006437609736487, -1.3336461209741413, -0.017833549159850304], [0.35855770640942686, 1.8571434623079024, -1.4041148558396288, -0.020755845044606074], [0.4114652020285343, 2.0139473340600365, -0.1937946219538823, -0.02382442826394008], [0.3499301521182933, 1.3389264069092857, -0.21029767748849823, -0.022723031905148013], [0.38059424489364246, 1.5220229333510222, -0.1302571590494475, -0.016263248981750543], [0.4207868671061959, 1.9890909149992932, -0.11465078250135777, -0.019859715040226194], [0.4148040618017305, 1.6458278151709658, -0.41822866513797036, -0.02596361679279958]], [[0.2938047023063933, 0.15848081496267857, 0.21377935785301977, -0.017044009015294515], [0.3578200533394036, 1.440800298674786, -0.25425224089524223, -0.013068948485870282], [0.35091888359219314, 1.346093085991901, 0.03700652414677099, -0.018437088761087322], [0.2615412035983308, 0.2553357946660699, 0.06563804987560529, -0.013729022790036183], [0.27744688808915585, 0.16285376720024541, 0.3969513138143117, -0.024167766761933995], [0.2410317694018692, 0.01719906807802845, 0.31887980936003024, -0.013899480418623898], [0.32670519203836695, 0.7070294256236573, 0.06889024493523768, -0.013849213382843669], [0.26929735820100886, 0.21585137293623718, 0.16764603161195335, -0.017509725152931335]], [[0.23964527052154094, 1.405161828042007, 0.7263938040790185, -0.013558480972783012], [0.23329678829132916, 1.9842641685831914, -0.43751729409466744, -0.009372812399959492], [0.29609136804454006, 2.2197331529484727, -0.3606187984687732, -0.014591349298057148], [0.18364046988106897, 1.0318842702071733, -0.21467102230538426, -0.006974976860324521], [0.237430149883509, 1.1354461619807799, 1.253426813991111, -0.010764567951424628], [0.21428788494745543, 1.2084708667209956, 0.6454519731653344, -0.014856742787382637], [0.19128550557336332, 0.9914202026492045, -0.012966520111932736, -0.01039845002841516], [0.18478085458589122, 0.6855671795600868, -0.05129936188141995, -0.014242565681526993]], [[0.15123693469828958, 1.163110201653609, 0.8745656657567553, -0.006604690732614436], [0.1617626592665295, 1.8451285513720417, -0.22859918528260925, -0.006219911053321165], [0.16565366259007014, 1.6280136877205398, -0.10883101331753334, -0.00964042687757254], [0.10928971110762957, 0.749493310399407, 0.003138228221609993, -0.008573046658971014], [0.02253022817352303, 0.07522041477715277, 0.8174746482416958, -0.007898334309960686], [0.003821773667235064, 0.19087983139285825, 1.2250839805129892, -0.006940107606339307], [0.17999809793891175, 1.4975328046377405, -0.11799490261557272, -0.0031203973369017474], [0.12067298238529153, 0.8183571646791823, 0.21700018598403456, -0.003330307143816533]], [[-0.0005213232213452705, 0.11664433274256322, -0.14703000948528538, 0.0022223370156425545], [-0.004751436308695322, 0.44945437865127735, 0.4407582496415892, 0.0009313311130397984], [-0.04601125513680242, 0.12232865474884935, -0.5555144671157969, -0.008711753743847687], [0.0, 0.0, 0.0, 0.0], [-0.0006907142392795103, 0.0644444433024974, -0.0722068891602118, -0.0030870140283082302], [0.001947573415548731, 0.009430552383996885, 0.376950878453279, 0.004011208280281968], [0.00601799297429685, -0.171200104000229, 0.4028188227208616, -0.0006892635684963884], [-0.0035595026932949752, -0.1639845558444737, 0.20081933970234833, 0.0007759675622934727]], [[-0.0445905899107714, 0.3878308646235794, 0.2999945087607148, 0.0006132606194773083], [-0.0233479900245816, 0.805464715742334, 0.002260800741456181, 0.0007923205997293554], [-0.027075628767392633, 0.21947910469952261, -0.6085871209249598, -0.00044238879126859074], [-0.14801341061316545, -0.9604402676156238, 0.04927742722480564, -0.010081622437758307], [-0.1351946090418747, -1.4037614517100776, 0.19096669008196027, -0.0005919410201843423], [-0.025443865945330033, 0.16995044160417527, -0.1562744263326309, -0.00198507171588911], [-0.017148669006657007, 0.20096477942386526, -0.0948436802257652, -0.0037168132796431656], [-0.045635057561963205, -0.07042763819321216, 0.178354420444418, -0.001384743167300897]], [[-0.14847892629844361, -2.1190919588657353, -0.39668969526474496, -0.003525009441780651], [-0.15170487526883455, -1.517780253977753, 0.40100295859357254, -0.003671659512345847], [-0.15582312230276163, -1.749691739278918, 0.4041461560506011, -0.006519857435921785], [-0.1490680046293541, -2.141748665352092, 0.4764301961883949, -0.0037233647798519207], [-0.19546209831376074, -3.094433551917896, 0.10995617619126552, -0.0013108345240767923], [-0.1663997352333837, -2.5234347104959314, 0.016952984209117655, -0.001558016324829012], [-0.16864610100772026, -2.2519891134627716, 0.009421852652772325, -0.0015948467476679916], [-0.17038719997008178, -2.6042474433647995, 0.09965476021822894, -0.0009880362442417799]], [[-0.1917409778980073, -3.892103482576627, 0.011307393107903144, -0.000973113351354111], [-0.23155366010446854, -3.73698000173536, -0.32159229488976254, 0.0043611241773148105], [-0.2149861492875637, -3.826512088064914, 0.35988121969000053, -0.003276087734406148], [-0.1850914206691932, -3.9073215173591516, -0.2976902305965188, 0.0018181088617474789], [-0.2166956185114457, -4.759035950022652, -0.39731132566536975, -0.0018975172421048176], [-0.18453416290159624, -4.081079332925176, 0.06634914312032889, 0.007699054345041634], [-0.18380968001623293, -3.94398458212836, 0.05540268327058757, 0.0077636042799711326], [-0.17894442370330435, -4.023445572474, 0.174749370962602, 0.005127314289389062]], [[-0.2071791595959074, -5.602941921550978, 0.5697348661401064, -0.004793728154630928], [-0.293851025233213, -6.076200837157158, 0.36633789088880986, -0.014666619442646871], [-0.3125311419595355, -6.474337848680638, -0.46570696369851816, -0.012047430951543585], [-0.2759968219061918, -6.572782260152643, 0.26886806477602143, -0.012852068603061987], [-0.2936587113768818, -6.974886539171132, 0.8883198818115932, -0.012730943822099026], [-0.23093202328582216, -6.1827075386667865, 0.9316427529555751, -0.012210883924464684], [-0.28464868233601415, -6.72909589800129, -0.19611855518100219, -0.00903527061959048], [-0.2625995405221107, -6.8102546031636955, 0.02108551835502591, -0.015084825328907772]], [[-0.017109063375111363, -6.305395147464962, 0.8493065447613946, -0.0027315707279580337], [-0.025183233654072573, -5.719115295608953, 0.25604355824758657, -0.0008328457993723413], [-0.011810426477860672, -5.756876322861796, 0.037077228631617845, -0.00508825489568598], [-0.021815470429823007, -6.764253867141102, 0.7528849605016921, -0.001718709211005901], [-0.017242461928480585, -6.867507311676377, 1.2998216029802259, -0.003178406222625727], [-0.1367473207454842, -7.368894585862941, 1.2187395147519533, 0.0011206638129489343], [-0.13939835532615258, -7.51839746503113, -0.16250224198741448, -0.008004712668605848], [-0.019153970264270632, -7.0125243850261025, 1.3284409701928372, -0.004219811523833364]], [[0.019682306949207716, -8.419884602382986, 0.6732033220764355, 0.0015869408442581077], [0.1342676842136754, -7.524039725140825, -0.37431134795767795, 0.003773576453475305], [0.1314848286265471, -7.858634951598969, 0.4067984956167212, -0.00041680645119449424], [-0.0023769326802557484, -9.435599598027125, 0.04226250370073082, -0.0045766590234569745], [0.11415934582312011, -8.967065961888935, 1.1616912507982886, 0.0017424276137151474], [0.006886096932619226, -9.124538610282109, 1.3445567104771639, 0.0021914730965736707], [0.0011853546556687636, -9.42889296285466, -0.09425767127590956, 0.004899855600506488], [-0.0031300437858024876, -9.620240941440606, -0.02985151339072315, -0.0035285519984824773]], [[0.19158100537043612, -9.973878447787747, -0.006863624293562527, -0.005091277194434075], [0.26447987114487426, -8.724786342424533, -0.07774075287962218, -0.004724860309786319], [0.1996364939410272, -9.360313632123415, -0.8082526536375445, -0.0056144966941685925], [0.2084764480893021, -10.169127800537426, -0.03308889327708536, -0.002301697763028448], [0.2372275579557133, -10.250819861501277, -0.056431256502948675, -0.0038013832607461037], [0.1922509036033489, -10.281680271187199, -0.16106822688380604, -0.0038161217587472586], [0.20343667754654882, -10.455658775951685, 0.04638001027351282, 0.0004225148653823805], [0.20924605109911876, -10.645286383709237, -0.2560681558188696, -0.009009170704748135]], [[0.8324350254386008, -7.5738976594623715, 0.014329030602573734, 0.006901506367214101], [0.8319769111866963, -7.325862948770705, -0.8312681835893114, 0.010517963078141769], [0.8353323200023774, -7.535011597070012, -1.3023747225436964, 0.0021814193999445996], [0.8316841554801186, -8.243511372338293, 0.0007712661209171201, 0.004297280031524099], [0.8325965528064283, -8.383550047857502, 0.07709444913444323, 0.0065460209544277795], [0.8801192911648763, -7.647708169014859, 0.16465071042293827, 0.004311475678621823], [0.9081305422228638, -7.550188011285636, 0.06288874368262504, 0.007952893331817507], [0.7179312827937098, -9.41628946575151, -0.14327709681944711, 0.0048404562595646735]]]
  in  "3D config":T1={"xyz pos"=[100, 67, 32], "color 4"={"color array"=[0, 8388736, 16711680, 16776960, 16776960, 16711680, 16448250, 16448250], "num of colors"=4, "max"=7000.900000000023, "min"=110.0}, "autogain"=TRUE, "zoom"=1.0, "slice(T)/stack(F)"=FALSE, "xy cut mag"=1.0330000000000057, "xy cut ofst"=-31.0, "z/xy comp"=0.9999999999999994, "y shift comp"=0.0, "max plot"=TRUE, "oblique angle [deg]"=45.0, "voxel size z [um]"=1.2257412881585255, "voxel size xy[um]"=0.455, "reverse v"=FALSE, "reverse h"=TRUE, "3D reconstruction"=TRUE, "reverse z"=FALSE} {"oblique angle [deg]" format="%_4g"; "y shift comp" format="%_4g"; "z/xy comp" format="%_4g"; "xy cut mag" format="%_4g"; "zoom" format="%_3g"; "color 4"."min" step=0.01 format="%_2f"; "color 4"."max" step=0.1 format="%_3f"}
  out "Timestamp":dbl=258.8159189224243
  out "rec start":bool
  in  "use most recent":bool=TRUE
  out "error out 2":errorcluster
  in  "config":T2={"Interpolation Type in"=0, "cam ofst"=100, "virtual slit center"=0.0, "virtual slit width ratio"=1.0, "overlay x"=607, "overlay y"=349, "BF pixel size"=1.152, "FL pixel size"=0.40900000000000003, "oblique angle"=45.0, "AOD scan speed ratio"=7.0, "Nx"=141.32142857142858, "y compensation"=0.0, "rotation [deg]"=0.0, "slice cut ofst"=0.0, "init pos mag"=1.0000000000000004, "slice cut mag"=1.0} {"slice cut mag" min=1e-05 format="%_4g"; "init pos mag" min=0.001; "rotation [deg]" format="%.2f"; "y compensation" format="%_4g"; "Interpolation Type in" items=["Zero Order", "Bi-Linear", "Quadratic", "Cubic Spline"]}
  in  "overlay FL to BF":bool=TRUE
  in  "slice cut pos":path=path "E:/calibration/20241014-04006.calib"
  out "folder name":string="20241014-00703zebrafish"
  in  "Zoom":sgl=0.70000005 format="%_3g"
  in  "color scale":T3={"colors 2"=[{"color array"=[0, 16448250, 16448250, 16448250, 16776960, 16711680, 16448250, 16448250], "num of colors"=2, "max"=255.0, "min"=130.0}, {"color array"=[0, 16711680, 16776960, 16448250, 16776960, 16711680, 16448250, 16448250], "num of colors"=4, "max"=30000.0, "min"=100.0}, {"color array"=[0, 16711680, 16448250, 16448250, 16776960, 16711680, 16448250, 16448250], "num of colors"=2, "max"=12500.0, "min"=0.0}, {"color array"=[0, 255, 16448250, 16448250, 16776960, 16711680, 16448250, 16448250], "num of colors"=2, "max"=1.01, "min"=0.0}, {"color array"=[0, 65280, 16448250, 16448250, 16776960, 16711680, 16448250, 16448250], "num of colors"=3, "max"=1.0, "min"=0.0}, {"color array"=[0, 255, 16448250, 16448250, 16776960, 16711680, 16448250, 16448250], "num of colors"=2, "max"=1.0099999999999991, "min"=0.0}], "on/off 2"=[TRUE, TRUE, FALSE, FALSE, FALSE, FALSE], "fast/slow"=FALSE, "on/off"=TRUE} {"colors 2"."min" step=0.01 format="%_2f"; "colors 2"."max" step=0.1 format="%_3f"}
  out "BF":picture
  out "Error Out":errorcluster caption="error"
  out "max value":u16=13141
  in  "color 2":T4={"color array"=[0, 16711680, 16776960, 16448250, 16776960, 16711680, 16448250, 16448250], "num of colors"=4, "max"=401.0, "min"=100.0, "auto"=TRUE, "Zoom"=0.6699995} {"Zoom" format="%_2g"; "min" step=0.01 format="%_2f"; "max" step=0.1 format="%_3f"}
  in  "master(F)/slave(T)":bool
  in  "one PC":bool=TRUE
  out "r-t time [s]":dbl=2.2499999886349542e-05
  in  "use global setting":bool=TRUE
  out "sCMOS":bool
  in  "frames to record":u32=10
  out "stop 2":bool=TRUE
  out "Numeric":i32=1190527
  out "timestamp intervals":dbl[](graph)=[0.006551980972290039, 0.006580829620361328, 0.006547212600708008, 0.006580829620361328, 0.006546974182128906, 0.00658106803894043, 0.006551980972290039, 0.00658106803894043, 0.006546974182128906]
  in  "REC":bool
  in  "buffer frames":i32=10000
  out "Frame Count":i32=1018
  out "file index":i32=9
  in  "foldername header":string="zebrafish"
  in  "monitor":bool=TRUE
  out "SVW":i32=300
  out "SVO":i32=1008
  out "error out":errorcluster
  in  "stop":bool
  # "Cam2 V offset: 868"
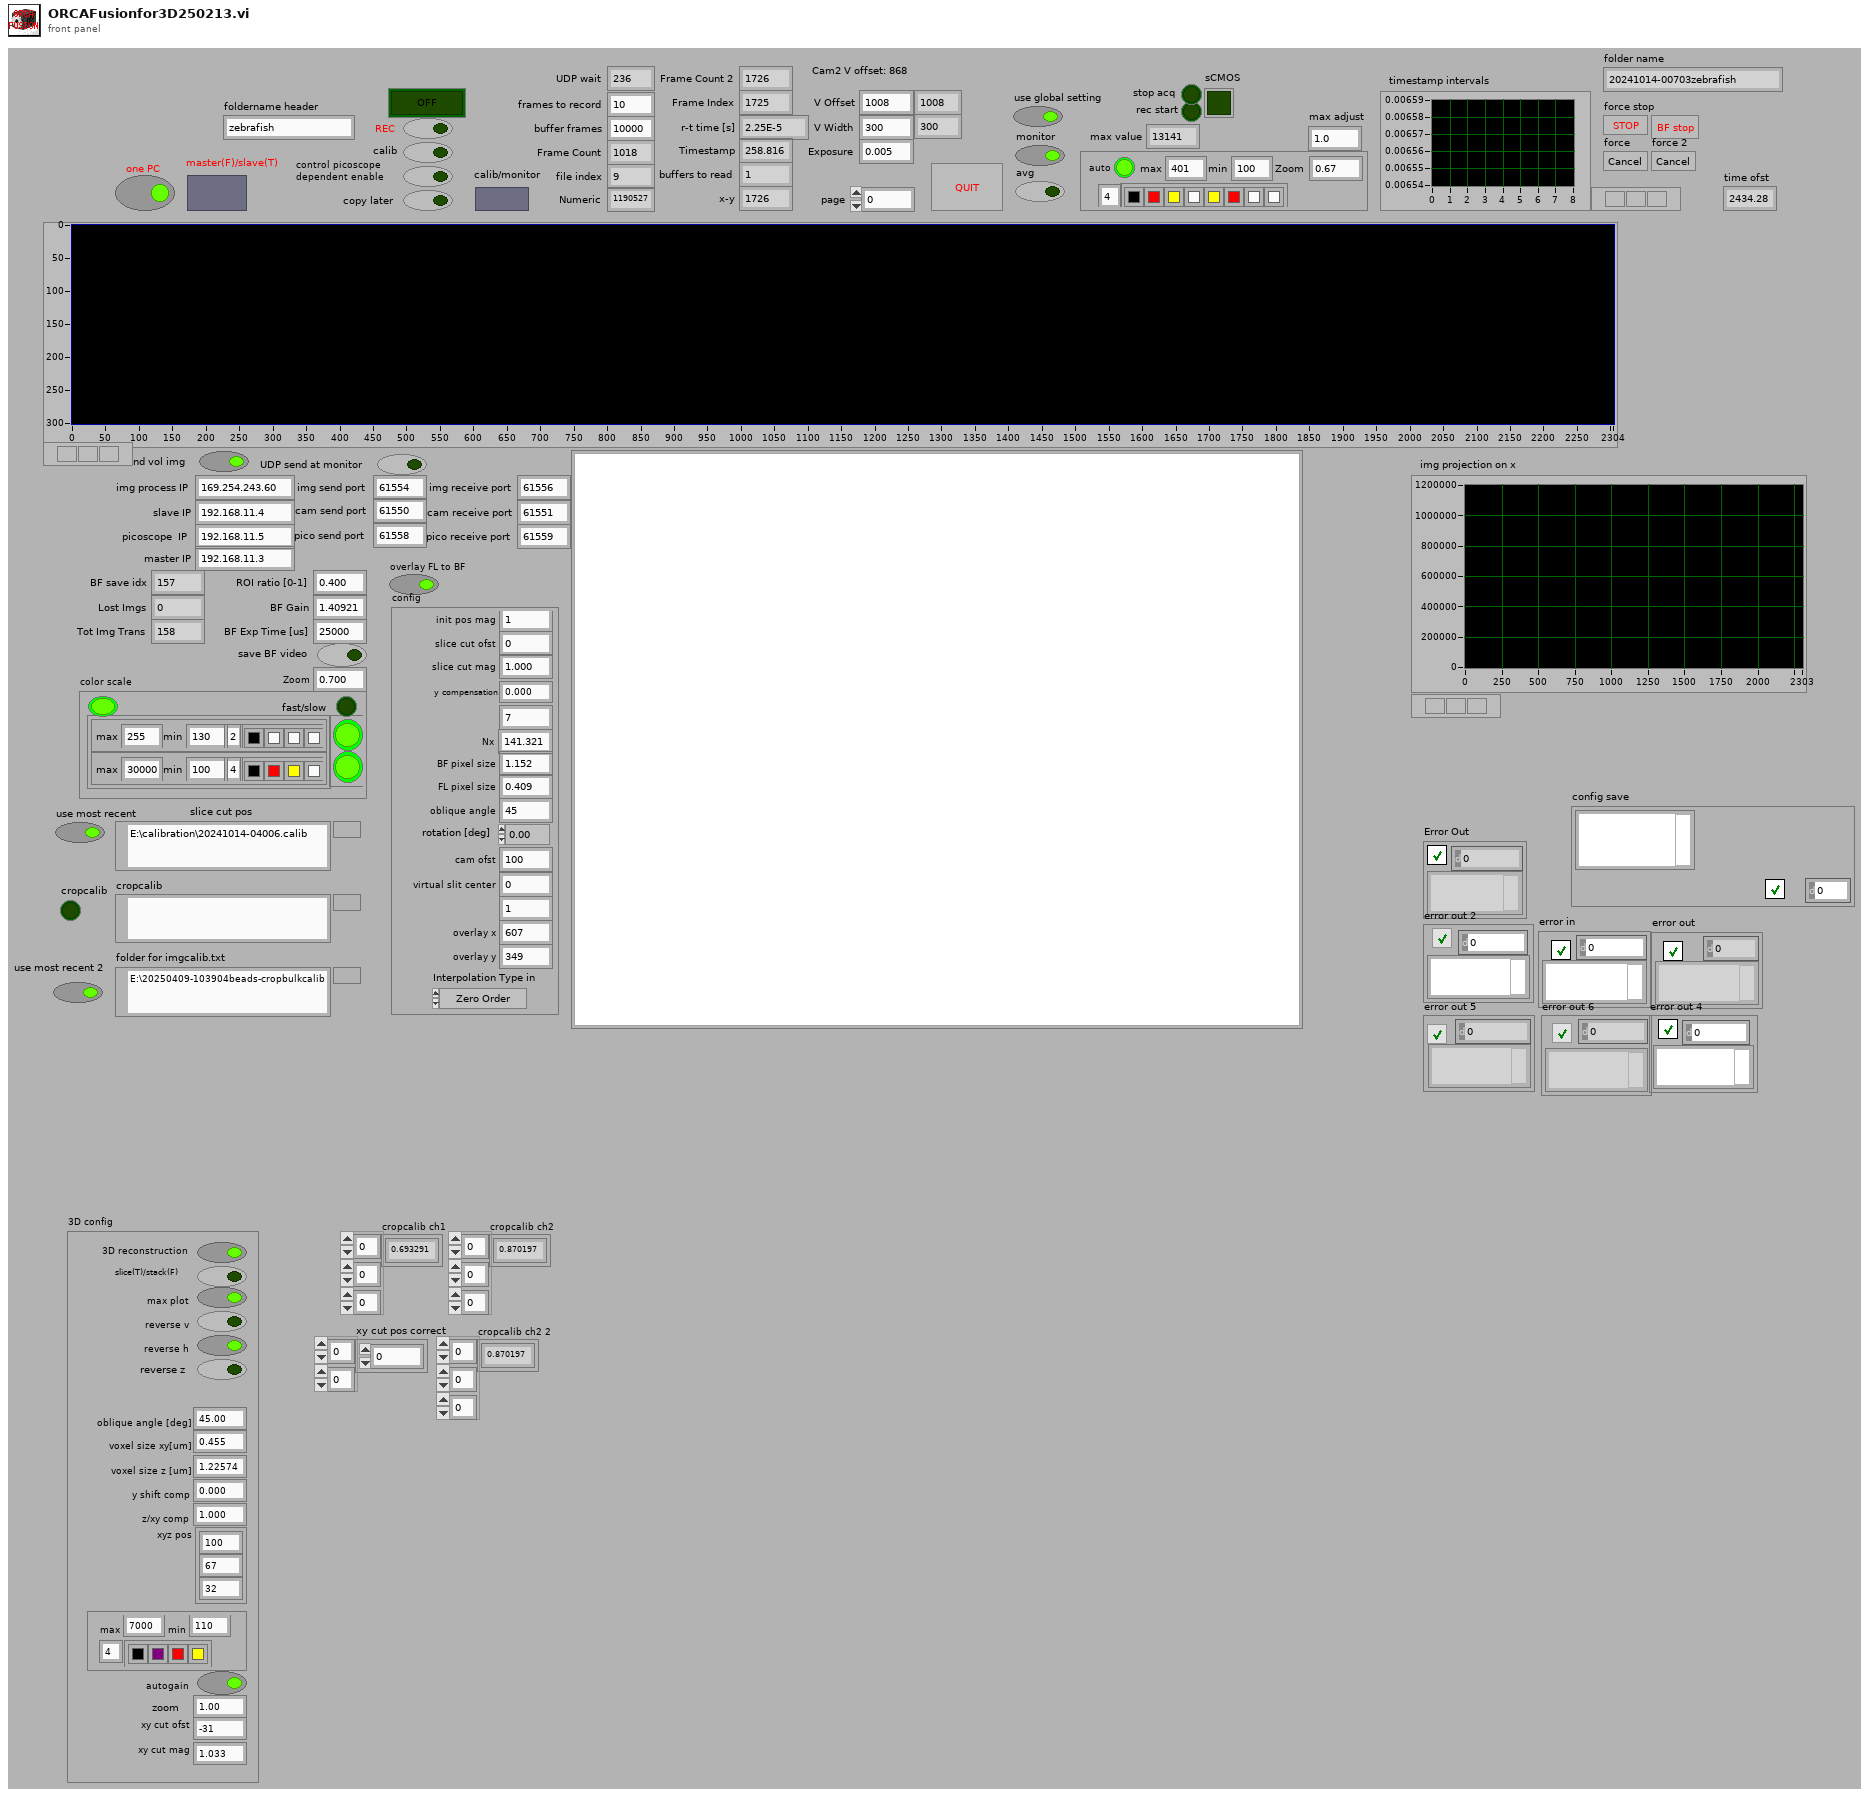
[diagram p1: front panel]
types:
  T1 = cluster{"xyz pos":u16[], "color 4":cluster{"color array":u32[], "num of colors":i32, "max":dbl, "min":dbl}, "autogain":bool, "zoom":dbl, "slice(T)/stack(F)":bool, "xy cut mag":dbl, "xy cut ofst":dbl, "z/xy comp":dbl, "y shift comp":dbl, "max plot":bool, "oblique angle [deg]":dbl, "voxel size z [um]":dbl, "voxel size xy[um]":dbl, "reverse v":bool, "reverse h":bool, "3D reconstruction":bool, "reverse z":bool}
  T2 = cluster{"Interpolation Type in":u32, "cam ofst":u16, "virtual slit center":dbl, "virtual slit width ratio":dbl, "overlay x":i32, "overlay y":i32, "BF pixel size":dbl, "FL pixel size":dbl, "oblique angle":dbl, "AOD scan speed ratio":dbl, "Nx":dbl, "y compensation":dbl, "rotation [deg]":sgl, "slice cut ofst":dbl, "init pos mag":dbl, "slice cut mag":dbl}
  T3 = cluster{"colors 2":cluster{"color array":u32[], "num of colors":i32, "max":dbl, "min":dbl}[], "on/off 2":bool[], "fast/slow":bool, "on/off":bool}
  T4 = cluster{"color array":u32[], "num of colors":i32, "max":dbl, "min":dbl, "auto":bool, "Zoom":sgl}
  T5 = cluster{"config cluster":cluster{"xy cut pos correct":dbl[][], "3D reconst config":cluster{"xyz pos":u16[], "color 4":cluster{"color array":u32[], "num of colors":i32, "max":dbl, "min":dbl}, "autogain":bool, "zoom":dbl, "slice(T)/stack(F)":bool, "xy cut mag":dbl, "xy cut ofst":dbl, "z/xy comp":dbl, "y shift comp":dbl, "max plot":bool, "oblique angle [deg]":dbl, "voxel size z [um]":dbl, "voxel size xy[um]":dbl, "reverse v":bool, "reverse h":bool, "3D reconstruction":bool, "reverse z":bool}, "xy cut pos":dbl[][], "AOD scan speed ratio":dbl, "Nx":dbl, "stack method":enum16{"0pad to z", "0pad to x", "0pad to x and rot"}, "y shift":i32}, "optimized param":dbl[][][][]}
  T6 = cluster{"img scan pos":dbl[][], "g1 disp [um]":dbl, "z spacing [um]":dbl, "g2 disp [pixels]":dbl, "scape scan pos ":dbl[]}
  T7 = cluster{"xy cut pos correct":dbl[][], "3D reconst config":cluster{"xyz pos":u16[], "color 4":cluster{"color array":u32[], "num of colors":i32, "max":dbl, "min":dbl}, "autogain":bool, "zoom":dbl, "slice(T)/stack(F)":bool, "xy cut mag":dbl, "xy cut ofst":dbl, "z/xy comp":dbl, "y shift comp":dbl, "max plot":bool, "oblique angle [deg]":dbl, "voxel size z [um]":dbl, "voxel size xy[um]":dbl, "reverse v":bool, "reverse h":bool, "3D reconstruction":bool, "reverse z":bool}, "xy cut pos":dbl[][], "AOD scan speed ratio":dbl, "Nx":dbl, "stack method":enum16{"0pad to z", "0pad to x", "0pad to x and rot"}, "y shift":i32}
  T8 = typedef "IMAQdx.ctl" = refnum<k21>
  T9 = enum16{"0pad to z", "0pad to x", "0pad to x and rot", "none"}
  T10 = cluster{"xy cut pos correct":dbl[][], "3D reconst config":cluster{"xyz pos":u16[], "color 4":cluster{"color array":u32[], "num of colors":i32, "max":dbl, "min":dbl}, "autogain":bool, "zoom":dbl, "slice(T)/stack(F)":bool, "xy cut mag":dbl, "xy cut ofst":dbl, "z/xy comp":dbl, "y shift comp":dbl, "max plot":bool, "oblique angle [deg]":dbl, "voxel size z [um]":dbl, "voxel size xy[um]":dbl, "reverse v":bool, "reverse h":bool, "3D reconstruction":bool, "reverse z":bool}, "xy cut pos":dbl[][], "AOD scan speed ratio":dbl, "Nx":dbl, "stack method":enum16{"0pad to z", "0pad to x", "0pad to x and rot", "none"}, "y shift":i32}
  T11 = cluster{"H Offset":i32, "V Offset":i32, "H Width":i32, "V Width":i32}
  T12 = typedef "LVMinMaxIncTypeDef.ctl" = cluster{"Minimum":dbl, "Maximum":dbl, "Increment":dbl}
  T13 = cluster{"H Offset":cluster{"Value":i32, "Limits":T12}, "V Offset":cluster{"Value":i32, "Limits":T12}, "H Size":cluster{"Value":i32, "Limits":T12}, "V Size":cluster{"Value":i32, "Limits":T12}}
  T14 = typedef "IMAQ Image.ctl" = refnum<image>
  T15 = cluster{"g2 period [us]":dbl, "frames to record":u32, string}
  T16 = enum32{"Bad", "Idle", "Run top level", "Running"}
  T17 = enum16{"open", "replace", "create", "open or create", "replace or create", "replace or create with confirmation"}
  T18 = typedef "NI_Vision_Acquisition_Software.lvlib/IMAQdx Acquisition Mode.ctl" = enum32{"One Shot", "Continuous"}
  T19 = cluster{"File Type":string, "Quality":u32, "Compress":bool, "Lossless":bool, "Ratio":sgl, "Codec":string, "Frame Rate":u32, "Limit Frames":bool, "Max Frames":u32}
  T20 = typedef "NI_Vision_Acquisition_Software.lvlib/IMAQdx Buffer Number Mode.ctl" = enum32{"Next", "Last", "Buffer Number", "Every", "Last New"}
  T21 = typedef "imagedata.ctl" = cluster{"image type":i32, "image depth":i32, "image":u8[], "mask":u8[], "colors":u32[], "Rectangle":cluster{"left":i16, "top":i16, "right":i16, "bottom":i16}}
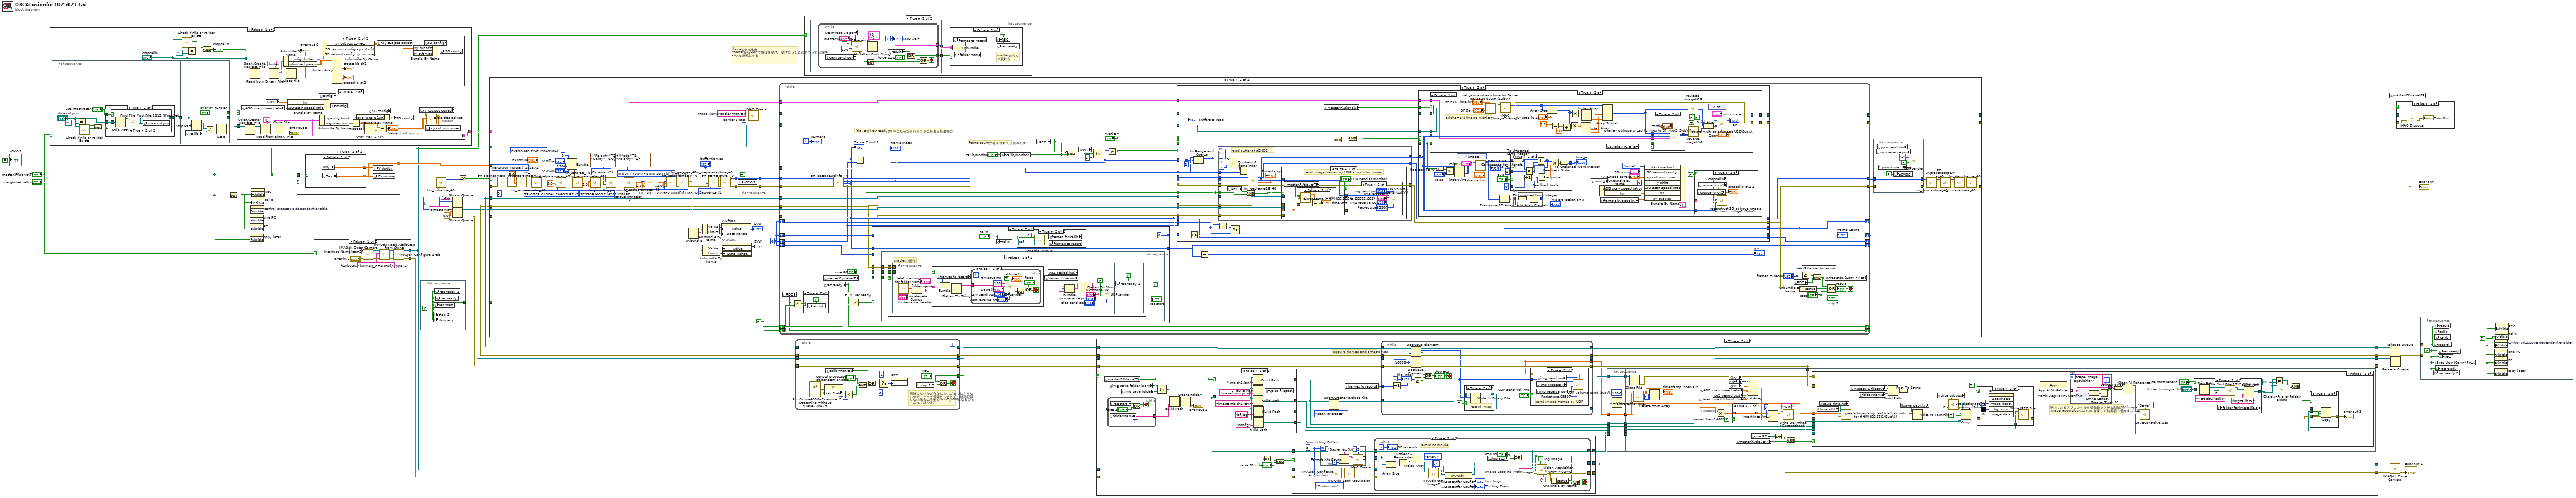
[diagram p0: block diagram]
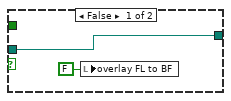
[diagram p7: hidden frame]
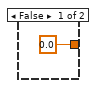
[diagram p11: hidden frame]
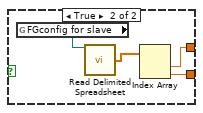
[diagram p12: hidden frame]
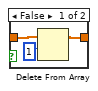
[diagram p15: hidden frame]
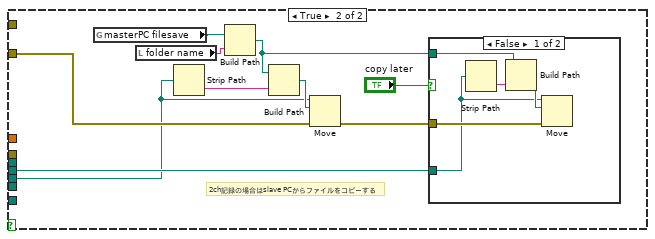
[diagram p19: hidden frame]
diagram:
  # "slaveのみの動作\nmasterからUDPで情報を受け、受け取ったことをもって記録readyな状態にする"
  n1 = case shown="False" "master(F)/slave(T)" {
    tunnel: [w46 _] -> w11
    frame False {
      n2 = flat-sequence {
        tunnel: [w65] -> w44
        tunnel: [w83] -> w45
        tunnel: w44 -> [w83]
        tunnel: ["overlay FL to BF"] -> w43
        frame #0 {
          n3 = Not Equal?(x="slice cut pos", y=path "" ("source path 3")) -> (x != y?=w68:bool)
          n4 = call <vilib>:"Check if File or Folder Exists.vi"("path"="slice cut pos") -> ("file or folder exists?"=w69:bool)  [unwired: 8 in, 2 out]
          n5 = And(x=w68, y=w69) -> (x .and. y?=w67:bool)
          n6 = case shown="True" w67 {
            tunnel: "slice cut pos" -> [w71 w75]
            tunnel: [w71 w74] -> w65
            tunnel: "use most recent" -> [_ w73]
            frame False {
              n7 = local write "overlay FL to BF"(FALSE) -> ()
            }
            frame True {
              n8 = case shown="True" w73 {
                tunnel: w75 -> [w76 w78]
                tunnel: [w76 w77] -> w74
                frame False {
                }
                frame True {
                  n9 = Strip Path(path=w78) -> (stripped path=w79:path)  [unwired: 1 out]
                  n10 = call "Find The Most File 2012 NIVerified.vi"("Folder Path In"=w79) -> ("File Path Out"=w77:path)  [unwired: 9 in, 1 out]
                  n11 = local write "slice cut pos"(w77) -> ()
                }
              }
            }
          }
        }
        frame #1 {
          n12 = global read "filepath global variable.vi" ".calib"() -> (w81:path)
          n13 = Strip Path(path=w83) -> (stripped path=w82:path)  [unwired: 1 out]
          n14 = Not Equal?(x=w82, y=w81) -> (x != y?=w80:bool)
          n15 = Stop(stop? (T)=w80) -> ()
        }
      }
      n16 = call <vilib>:"Check if File or Folder Exists.vi"("path"="cropcalib") -> ("file or folder exists?"=w39:bool)  [unwired: 8 in, 2 out]
      n17 = Not Equal?(x="cropcalib", y=path "" ("source path 3")) -> (x != y?=w38:bool)
      n18 = And(x=w39, y=w38) -> (x .and. y?=w40:bool)
      "cropcalib" <- w40
      n19 = case shown="True" w43 {
        tunnel: [_ w90] -> w46
        tunnel: w45 -> [_ w98]
        frame False {
        }
        frame True {
          n20 = global read "global for picoscope.vi" "AOD scan speed ratio"() -> (w99:dbl)
          n21 = Open/Create/Replace File(file path (use dialog)=w98) -> (refnum out=w102:refnum<file>, error out=w101:errorcluster)  [unwired: 5 in, 1 out]
          n22 = Read from Binary File(5:T6 {"img scan pos"=[], "g1 disp [um]"=0.0, "z spacing [um]"=0.0, "g2 disp [pixels]"=0.0, "scape scan pos "=[]} ("output cluster 2"), 8:w101, 11:w102) -> (0:w105:errorcluster, 2:w90:T6, 3:w104:refnum<file>)  [unwired: 3 in, 1 out]
          n23 = global read "global for picoscope.vi" "Nx"() -> (w100:dbl)
          n24 = Close File(refnum=w104, error in=w105) -> (error out=→"error out 5":errorcluster)  [unwired: 1 out]
          n25 = local read "config"() -> (w97:T2)
          n26 = Bundle By Name(cluster=w97, "Nx"=w100, "AOD scan speed ratio"=w99) -> (w96:T2)
          n27 = Unbundle By Name(w90) -> ("z spacing [um]"=w93:dbl, "img scan pos"=w92:dbl[][])
          n28 = local write "config"(w96) -> ()
          n29 = Negate(x=w92) -> (-x=w91:dbl[][])
          n30 = Array Max & Min(array=w91) -> (min value=w95:dbl)  [unwired: 3 out]
          n31 = local read "3D config"() -> (w87:T1)
          n32 = Bundle By Name(cluster=w87, "voxel size z [um]"=w93) -> (w86:T1)
          n33 = Subtract(x=w91, y=w95) -> (x-y=w94:dbl[][])
          "frame's init pos in x" <- w94
          n34 = local write "3D config"(w86) -> ()
          n35 = local read "xy cut pos correct"() -> (w89:dbl[][])
          n36 = call "table size adjust (SubVI).vi"("Array in"=w94, "xy cut pos correct"=w89) -> ("Array out"=w88:dbl[][])  [unwired: 9 in]
          n37 = local write "xy cut pos correct"(w88) -> ()
        }
      }
      n38 = case shown="True" w40 {
        tunnel: "cropcalib" -> [_ w60]
        frame False {
        }
        frame True {
          n39 = Open/Create/Replace File(file path (use dialog)=w60) -> (refnum out=w59:refnum<file>, error out=w63:errorcluster)  [unwired: 5 in, 1 out]
          n40 = Read from Binary File(5:T5 {"config cluster"={"xy cut pos correct"=[], "3D reconst config"={"xyz pos"=[], "color 4"={"color array"=[], "num of colors"=0, "max"=0.0, "min"=0.0}, "autogain"=FALSE, "zoom"=0.0, "slice(T)/stack(F)"=FALSE, "xy cut mag"=0.0, "xy cut ofst"=0.0, "z/xy comp"=0.0, "y shift comp"=0.0, "max plot"=FALSE, "oblique angle [deg]"=0.0, "voxel size z [um]"=0.0, "voxel size xy[um]"=0.0, "reverse v"=FALSE, "reverse h"=FALSE, "3D reconstruction"=FALSE, "reverse z"=FALSE}, "xy cut pos"=[], "AOD scan speed ratio"=0.0, "Nx"=0.0, "stack method"=enum."0pad to z", "y shift"=0}, "optimized param"=[]} ("cluster"), 8:w63, 11:w59) -> (0:w62:errorcluster, 2:w57:T5, 3:w61:refnum<file>)  [unwired: 3 in, 1 out]
          n41 = Unbundle By Name(w57) -> ("config cluster"=w53:T7, "optimized param"=w56:dbl[][][][])
          n42 = Close File(refnum=w61, error in=w62) -> (error out=→"error out 6":errorcluster)  [unwired: 1 out]
          n43 = Unbundle By Name(w53) -> ("xy cut pos correct"=w48:dbl[][], "3D reconst config.xy cut ofst"=w52:dbl, "3D reconst config.xy cut mag"=w51:dbl)
          n44 = Index Array(array=w56) -> (element #1=→"cropcalib ch1":dbl[][][], element #2=→"cropcalib ch2":dbl[][][])  [unwired: 8 in]
          n45 = local write "xy cut pos correct"(w48) -> ()
          n46 = local read "3D config"() -> (w50:T1)
          n47 = Bundle By Name(cluster=w50, "xy cut ofst"=w52, "xy cut mag"=w51) -> (w49:T1)
          n48 = local write "3D config"(w49) -> ()
        }
      }
    }
    frame True {
    }
  }
  n49 = Not(x="master(F)/slave(T)") -> (.not. x?=w1:bool)
  n50 = property on="one PC" class="Bool (strict)"("Visible"=w1) -> ()  [unwired: 2 in, 2 out]
  n51 = property on="BF" class="Pict"("Visible"=w1) -> ()  [unwired: 2 in, 2 out]
  n52 = property on="copy later" class="Bool (strict)"("Visible"="master(F)/slave(T)") -> ()  [unwired: 2 in, 2 out]
  n53 = property on="control picoscope dependent enable" class="Bool (strict)"("Visible"=w1) -> ()  [unwired: 2 in, 2 out]
  n54 = property on="calib" class="Bool (strict)"("Visible"=w1) -> ()  [unwired: 2 in, 2 out]
  n55 = property on="REC" class="Bool (strict)"("Visible"=w1) -> ()  [unwired: 2 in, 2 out]
  n56 = case shown="True" "use global setting" {
    tunnel: [0.0 ("Tex") w107] -> w23
    tunnel: "master(F)/slave(T)" -> [_ w109]
    frame False {
    }
    frame True {
      n57 = case shown="False" w109 {
        tunnel: [w111 w113] -> w107
        tunnel: [w110 w114] -> w108
        frame False {
          n58 = global read "Global for awg.vi" "Ny"() -> (w110:dbl)
          n59 = global read "Global for awg.vi" "Tex"() -> (w111:dbl)
        }
        frame True {
          n60 = global read "filepath global variable.vi" "FGconfig for slave"() -> (w112:path)
          n61 = call-poly <vilib>:"Read Delimited Spreadsheet.vi"("file path (dialog if empty)"=w112) -> ("first row"=w115:dbl[])  [unwired: 9 in, 5 out]
          n62 = Index Array(array=w115) -> (element #1=w114:dbl, element #2=w113:dbl)  [unwired: 2 in]
        }
      }
      n63 = local write "Exposure"(w107) -> ()
      n64 = local write "V Width"(w108) -> ()
    }
  }
  n65 = case shown="False" "master(F)/slave(T)" {
    tunnel: [w117 _] -> w9
    tunnel: [w116 _] -> w5
    frame False {
      w118 = "[NIIMAQ_HEADER]\nType = 2\nVersion = 8\n\n[CAMERA_DATA]\nAcquisitionAttributes::AdvancedGenicam::CommandTimeout = \"100\"\nAcquisitionAttributes::AdvancedGenicam::EventQueueDepth = \"50\"\nAcquisitionAttributes::AdvancedGenicam::EventsEnabled = \"true\"\nAcquisitionAttributes::AdvancedGenicam::IgnoreCameraValidationErrors = \"false\"\nAcquisitionAttributes::AdvancedGenicam::PersistenceAlgorithm = \"Auto\"\nAcquisitionAttributes::AdvancedUSB3Vision::DesiredMaximumPayloadTransferSize = \"4294967295\"\nAcquisitionAttributes::Bayer::Algorithm = \"Bilinear\"\nAcquisitionAttributes::Bayer::GainB = \"1\"\nAcquisitionAttributes::Bayer::GainG = \"1\"\nAcquisitionAttributes::Bayer::GainR = \"1\"\nAcquisitionAttributes::Bayer::Pattern = \"Use hardware value\"\nAcquisitionAttributes::BitsPerPixel = \"Use hardware value\"\nAcquisitionAttributes::ChunkDataDecoding::ChunkDataDecodingEnabled = \"false\"\nAcquisitionAttributes::ChunkDataDecoding::MaximumChunkCopySize = \"64\"\nAcquisitionAttributes::HardwareMaximumQueuedBufferCount = \"1000\"\nAcquisitionAttributes::HardwareRequeueBufferListThreshold = \"50\"\nAcquisitionAttributes::IgnoreFirstFrame = \"false\"\nAcquisitionAttributes::ImageDecoderCopyMode = \"Auto\"\nAcquisitionAttributes::IncompleteBufferMode = \"Ignore\"\nAcquisitionAttributes::OutputImageType = \"Auto\"\nAcquisitionAttributes::OverwriteMode = \"Get Newest\"\nAcquisitionAttributes::PixelSignedness = \"Use hardware value\"\nAcquisitionAttributes::ReceiveTimestampMode = \"None\"\nAcquisitionAttributes::ShiftPixelBits = \"false\"\nAcquisitionAttributes::SwapPixelBytes = \"false\"\nAcquisitionAttributes::Timeout = \"5000\"\nCameraAttributes::AcquisitionControl::ExposureAuto = \"Off\"\nCameraAttributes::AnalogControl::GainAuto = \"Off\"\nCameraAttributes::ImageFormatControl::Width = \"2592\"\nCameraAttributes::ImageFormatControl::Height = \"2048\"\nCameraAttributes::ImageFormatControl::OffsetX = \"0\"\nCameraAttributes::ImageFormatControl::OffsetY = \"0\"\nCameraAttributes::ImageFormatControl::CenterX = \"0\"\nCameraAttributes::ImageFormatControl::CenterY = \"0\"\nCameraAttributes::ImageFormatControl::BinningHorizontalMode = \"Average\"\nCameraAttributes::ImageFormatControl::BinningHorizontal = \"1\"\nCameraAttributes::ImageFormatControl::BinningVerticalMode = \"Average\"\nCameraAttributes::ImageFormatControl::BinningVertical = \"1\"\nCameraAttributes::ImageFormatControl::ReverseX = \"0\"\nCameraAttributes::ImageFormatControl::ReverseY = \"0\"\nCameraAttributes::ImageFormatControl::PixelFormat = \"Mono8\"\nCameraAttributes::ImageFormatControl::TestImageSelector = \"Off\"\nCameraAttributes::ImageFormatControl::ROIZoneSelector = \"Zone0\"\nCameraAttributes::ImageFormatControl::ROIZoneMode = \"Off\"\nCameraAttributes::ImageFormatControl::ROIZoneSelector = \"Zone1\"\nCameraAttributes::ImageFormatControl::ROIZoneMode = \"Off\"\nCameraAttributes::ImageFormatControl::ROIZoneSelector = \"Zone2\"\nCameraAttributes::ImageFormatControl::ROIZoneMode = \"Off\"\nCameraAttributes::ImageFormatControl::ROIZoneSelector = \"Zone3\"\nCameraAttributes::ImageFormatControl::ROIZoneMode = \"Off\"\nCameraAttributes::ImageFormatControl::ROIZoneSelector = \"Zone4\"\nCameraAttributes::ImageFormatControl::ROIZoneMode = \"Off\"\nCameraAttributes::ImageFormatControl::ROIZoneSelector = \"Zone5\"\nCameraAttributes::ImageFormatControl::ROIZoneMode = \"Off\"\nCameraAttributes::ImageFormatControl::ROIZoneSelector = \"Zone6\"\nCameraAttributes::ImageFormatControl::ROIZoneMode = \"Off\"\nCameraAttributes::ImageFormatControl::ROIZoneSelector = \"Zone7\"\nCameraAttributes::ImageFormatControl::ROIZoneMode = \"Off\"\nCameraAttributes::ImageFormatControl::ROIZoneSelector = \"Zone0\"\nCameraAttributes::ImageFormatControl::ROIZoneSelector = \"Zone0\"\nCameraAttributes::ImageFormatControl::ROIZoneSize = \"4\"\nCameraAttributes::ImageFormatControl::ROIZoneSelector = \"Zone1\"\nCameraAttributes::ImageFormatControl::ROIZoneSize = \"4\"\nCameraAttributes::ImageFormatControl::ROIZoneSelector = \"Zone2\"\nCameraAttributes::ImageFormatControl::ROIZoneSize = \"4\"\nCameraAttributes::ImageFormatControl::ROIZoneSelector = \"Zone3\"\nCameraAttributes::ImageFormatControl::ROIZoneSize = \"4\"\nCameraAttributes::ImageFormatControl::ROIZoneSelector = \"Zone4\"\nCameraAttributes::ImageFormatControl::ROIZoneSize = \"4\"\nCameraAttributes::ImageFormatControl::ROIZoneSelector = \"Zone5\"\nCameraAttributes::ImageFormatControl::ROIZoneSize = \"4\"\nCameraAttributes::ImageFormatControl::ROIZoneSelector = \"Zone6\"\nCameraAttributes::ImageFormatControl::ROIZoneSize = \"4\"\nCameraAttributes::ImageFormatControl::ROIZoneSelector = \"Zone7\"\nCameraAttributes::ImageFormatControl::ROIZoneSize = \"4\"\nCameraAttributes::ImageFormatControl::ROIZoneSelector = \"Zone0\"\nCameraAttributes::ImageFormatControl::ROIZoneSelector = \"Zone0\"\nCameraAttributes::ImageFormatControl::ROIZoneOffset = \"0\"\nCameraAttributes::ImageFormatControl::ROIZoneSelector = \"Zone1\"\nCameraAttributes::ImageFormatControl::ROIZoneOffset = \"0\"\nCameraAttributes::ImageFormatControl::ROIZoneSelector = \"Zone2\"\nCameraAttributes::ImageFormatControl::ROIZoneOffset = \"0\"\nCameraAttributes::ImageFormatControl::ROIZoneSelector = \"Zone3\"\nCameraAttributes::ImageFormatControl::ROIZoneOffset = \"0\"\nCameraAttributes::ImageFormatControl::ROIZoneSelector = \"Zone4\"\nCameraAttributes::ImageFormatControl::ROIZoneOffset = \"0\"\nCameraAttributes::ImageFormatControl::ROIZoneSelector = \"Zone5\"\nCameraAttributes::ImageFormatControl::ROIZoneOffset = \"0\"\nCameraAttributes::ImageFormatControl::ROIZoneSelector = \"Zone6\"\nCameraAttributes::ImageFormatControl::ROIZoneOffset = \"0\"\nCameraAttributes::ImageFormatControl::ROIZoneSelector = \"Zone7\"\nCameraAttributes::ImageFormatControl::ROIZoneOffset = \"0\"\nCameraAttributes::ImageFormatControl::ROIZoneSelector = \"Zone0\"\nCameraAttributes::AnalogControl::GainSelector = \"All\"\nCameraAttributes::AnalogControl::Gain = \"0.00000\"\nCameraAttributes::AnalogControl::GainSelector = \"All\"\nCameraAttributes::AnalogControl::BlackLevelSelector = \"All\"\nCameraAttributes::AnalogControl::BlackLevel = \"1.00000\"\nCameraAttributes::AnalogControl::BlackLevelSelector = \"All\"\nCameraAttributes::AnalogControl::Gamma = \"1.00000\"\nCameraAttributes::RemoveParameterLimitControl::RemoveParameterLimitSelector = \"Gain\"\nCameraAttributes::RemoveParameterLimitControl::RemoveParameterLimit = \"0\"\nCameraAttributes::RemoveParameterLimitControl::RemoveParameterLimitSelector = \"ExposureTime\"\nCameraAttributes::RemoveParameterLimitControl::RemoveParameterLimit = \"0\"\nCameraAttributes::RemoveParameterLimitControl::RemoveParameterLimitSelector = \"Gain\"\nCameraAttributes::ImageQualityControl::PGIControl::PgiMode = \"Off\"\nCameraAttributes::AcquisitionControl::ShutterMode = \"Global\"\nCameraAttributes::AcquisitionControl::ExposureMode = \"Timed\"\nCameraAttributes::AcquisitionControl::ExposureTime = \"5000.0\"\nCameraAttributes::AcquisitionControl::SensorReadoutMode = \"Normal\"\nCameraAttributes::AcquisitionControl::AcquisitionBurstFrameCount = \"1\"\nCameraAttributes::AcquisitionControl::TriggerSelector = \"FrameBurstStart\"\nCameraAttributes::AcquisitionControl::TriggerMode = \"Off\"\nCameraAttributes::AcquisitionControl::TriggerSelector = \"FrameStart\"\nCameraAttributes::AcquisitionControl::TriggerMode = \"Off\"\nCameraAttributes::AcquisitionControl::TriggerSelector = \"FrameStart\"\nCameraAttributes::AcquisitionControl::TriggerSelector = \"FrameBurstStart\"\nCameraAttributes::AcquisitionControl::TriggerSource = \"Line1\"\nCameraAttributes::AcquisitionControl::TriggerSelector = \"FrameStart\"\nCameraAttributes::AcquisitionControl::TriggerSource = \"Line1\"\nCameraAttributes::AcquisitionControl::TriggerSelector = \"FrameStart\"\nCameraAttributes::AcquisitionControl::TriggerSelector = \"FrameBurstStart\"\nCameraAttributes::AcquisitionControl::TriggerActivation = \"RisingEdge\"\nCameraAttributes::AcquisitionControl::TriggerSelector = \"FrameStart\"\nCameraAttributes::AcquisitionControl::TriggerActivation = \"RisingEdge\"\nCameraAttributes::AcquisitionControl::TriggerSelector = \"FrameStart\"\nCameraAttributes::AcquisitionControl::TriggerDelay = \"0\"\nCameraAttributes::AcquisitionControl::AcquisitionFrameRateEnable = \"1\"\nCameraAttributes::AcquisitionControl::AcquisitionFrameRate = \"25.00000\"\nCameraAttributes::DeviceControl::DeviceLinkSelector = \"0\"\nCameraAttributes::DeviceControl::DeviceLinkThroughputLimitMode = \"On\"\nCameraAttributes::DeviceControl::DeviceLinkSelector = \"0\"\nCameraAttributes::DeviceControl::DeviceLinkSelector = \"0\"\nCameraAttributes::DeviceControl::DeviceLinkThroughputLimit = \"300000000\"\nCameraAttributes::DeviceControl::DeviceLinkSelector = \"0\"\nCameraAttributes::ChunkDataControl::ChunkSelector = \"Gain\"\nCameraAttributes::ChunkDataControl::ChunkEnable = \"0\"\nCameraAttributes::ChunkDataControl::ChunkSelector = \"ExposureTime\"\nCameraAttributes::ChunkDataControl::ChunkEnable = \"0\"\nCameraAttributes::ChunkDataControl::ChunkSelector = \"Timestamp\"\nCameraAttributes::ChunkDataControl::ChunkEnable = \"0\"\nCameraAttributes::ChunkDataControl::ChunkSelector = \"LineStatusAll\"\nCameraAttributes::ChunkDataControl::ChunkEnable = \"0\"\nCameraAttributes::ChunkDataControl::ChunkSelector = \"CounterValue\"\nCameraAttributes::ChunkDataControl::ChunkEnable = \"0\"\nCameraAttributes::ChunkDataControl::ChunkSelector = \"SequencerSetActive\"\nCameraAttributes::ChunkDataControl::ChunkEnable = \"0\"\nCameraAttributes::ChunkDataControl::ChunkSelector = \"PayloadCRC16\"\nCameraAttributes::ChunkDataControl::ChunkEnable = \"0\"\nCameraAttributes::ChunkDataControl::ChunkSelector = \"Timestamp\"\nCameraAttributes::ChunkDataControl::ChunkModeActive = \"0\"\nCameraAttributes::AutoFunctionControl::AutoTargetBrightness = \"0.50196\"\nCameraAttributes::AutoFunctionControl::AutoFunctionProfile = \"MinimizeGain\"\nCameraAttributes::AutoFunctionControl::AutoGainLowerLimit = \"0.00000\"\nCameraAttributes::AutoFunctionControl::AutoGainUpperLimit = \"12.00920\"\nCameraAttributes::AutoFunctionControl::AutoExposureTimeLowerLimit = \"117.0\"\nCameraAttributes::AutoFunctionControl::AutoExposureTimeUpperLimit = \"500000.0\"\nCameraAttributes::AutoFunctionControl::AutoFunctionROIControl::AutoFunctionROISelector = \"ROI1\"\nCameraAttributes::AutoFunctionControl::AutoFunctionROIControl::AutoFunctionROIWidth = \"2592\"\nCameraAttributes::AutoFunctionControl::AutoFunctionROIControl::AutoFunctionROISelector = \"ROI2\"\nCameraAttributes::AutoFunctionControl::AutoFunctionROIControl::AutoFunctionROIWidth = \"2592\"\nCameraAttributes::AutoFunctionControl::AutoFunctionROIControl::AutoFunctionROISelector = \"ROI1\"\nCameraAttributes::AutoFunctionControl::AutoFunctionROIControl::AutoFunctionROISelector = \"ROI1\"\nCameraAttributes::AutoFunctionControl::AutoFunctionROIControl::AutoFunctionROIHeight = \"2048\"\nCameraAttributes::AutoFunctionControl::AutoFunctionROIControl::AutoFunctionROISelector = \"ROI2\"\nCameraAttributes::AutoFunctionControl::AutoFunctionROIControl::AutoFunctionROIHeight = \"2048\"\nCameraAttributes::AutoFunctionControl::AutoFunctionROIControl::AutoFunctionROISelector = \"ROI1\"\nCameraAttributes::AutoFunctionControl::AutoFunctionROIControl::AutoFunctionROISelector = \"ROI1\"\nCameraAttributes::AutoFunctionControl::AutoFunctionROIControl::AutoFunctionROIOffsetX = \"0\"\nCameraAttributes::AutoFunctionControl::AutoFunctionROIControl::AutoFunctionROISelector = \"ROI2\"\nCameraAttributes::AutoFunctionControl::AutoFunctionROIControl::AutoFunctionROIOffsetX = \"0\"\nCameraAttributes::AutoFunctionControl::AutoFunctionROIControl::AutoFunctionROISelector = \"ROI1\"\nCameraAttributes::AutoFunctionControl::AutoFunctionROIControl::AutoFunctionROISelector = \"ROI1\"\nCameraAttributes::AutoFunctionControl::AutoFunctionROIControl::AutoFunctionROIOffsetY = \"0\"\nCameraAttributes::AutoFunctionControl::AutoFunctionROIControl::AutoFunctionROISelector = \"ROI2\"\nCameraAttributes::AutoFunctionControl::AutoFunctionROIControl::AutoFunctionROIOffsetY = \"0\"\nCameraAttributes::AutoFunctionControl::AutoFunctionROIControl::AutoFunctionROISelector = \"ROI1\"\nCameraAttributes::AutoFunctionControl::AutoFunctionROIControl::AutoFunctionROISelector = \"ROI1\"\nCameraAttributes::AutoFunctionControl::AutoFunctionROIControl::AutoFunctionROIUseBrightness = \"1\"\nCameraAttributes::AutoFunctionControl::AutoFunctionROIControl::AutoFunctionROISelector = \"ROI2\"\nCameraAttributes::AutoFunctionControl::AutoFunctionROIControl::AutoFunctionROIUseBrightness = \"0\"\nCameraAttributes::AutoFunctionControl::AutoFunctionROIControl::AutoFunctionROISelector = \"ROI1\"\nCameraAttributes::AutoFunctionControl::AutoFunctionROIControl::AutoFunctionROISelector = \"ROI1\"\nCameraAttributes::AutoFunctionControl::AutoFunctionROIControl::AutoFunctionROIUseWhiteBalance = \"0\"\nCameraAttributes::AutoFunctionControl::AutoFunctionROIControl::AutoFunctionROISelector = \"ROI2\"\nCameraAttributes::AutoFunctionControl::AutoFunctionROIControl::AutoFunctionROIUseWhiteBalance = \"1\"\nCameraAttributes::AutoFunctionControl::AutoFunctionROIControl::AutoFunctionROISelector = \"ROI1\"\nCameraAttributes::LUTControl::LUTSelector = \"Luminance\"\nCameraAttributes::LUTControl::LUTEnable = \"0\"\nCameraAttributes::LUTControl::LUTSelector = \"Luminance\"\nCameraAttributes::LUTControl::LUTSelector = \"Luminance\"\nCameraAttributes::LUTControl::LUTValueAll = \"0x000000000000000002000000000000000400000000000000060000000000000008000000000000000a000000000000000c000000000000000e00000000000000100000000000000012000000000000001400000000000000160000000000000018000000000000001a000000000000001c000000000000001e00000000000000200000000000000022000000000000002400000000000000260000000000000028000000000000002a000000000000002c000000000000002e00000000000000300000000000000032000000000000003400000000000000360000000000000038000000000000003a000000000000003c000000000000003e00000000000000400000000000000042000000000000004400000000000000460000000000000048000000000000004a000000000000004c000000000000004e00000000000000500000000000000052000000000000005400000000000000560000000000000058000000000000005a000000000000005c000000000000005e00000000000000600000000000000062000000000000006400000000000000660000000000000068000000000000006a000000000000006c000000000000006e00000000000000700000000000000072000000000000007400000000000000760000000000000078000000000000007a000000000000007c000000000000007e00000000000000800000000000000082000000000000008400000000000000860000000000000088000000000000008a000000000000008c000000000000008e00000000000000900000000000000092000000000000009400000000000000960000000000000098000000000000009a000000000000009c000000000000009e00000000000000a000000000000000a200000000000000a400000000000000a600000000000000a800000000000000aa00000000000000ac00000000000000ae00000000000000b000000000000000b200000000000000b400000000000000b600000000000000b800000000000000ba00000000000000bc00000000000000be00000000000000c000000000000000c200000000000000c400000000000000c600000000000000c800000000000000ca00000000000000cc00000000000000ce00000000000000d000000000000000d200000000000000d400000000000000d600000000000000d800000000000000da00000000000000dc00000000000000de00000000000000e000000000000000e200000000000000e400000000000000e600000000000000e800000000000000ea00000000000000ec00000000000000ee00000000000000f000000000000000f200000000000000f400000000000000f600000000000000f800000000000000fa00000000000000fc00000000000000fe00000000000000000100000000000002010000000000000401000000000000060100000000000008010000000000000a010000000000000c010000000000000e01000000000000100100000000000012010000000000001401000000000000160100000000000018010000000000001a010000000000001c010000000000001e01000000000000200100000000000022010000000000002401000000000000260100000000000028010000000000002a010000000000002c010000000000002e01000000000000300100000000000032010000000000003401000000000000360100000000000038010000000000003a010000000000003c010000000000003e01000000000000400100000000000042010000000000004401000000000000460100000000000048010000000000004a010000000000004c010000000000004e01000000000000500100000000000052010000000000005401000000000000560100000000000058010000000000005a010000000000005c010000000000005e01000000000000600100000000000062010000000000006401000000000000660100000000000068010000000000006a010000000000006c010000000000006e01000000000000700100000000000072010000000000007401000000000000760100000000000078010000000000007a010000000000007c010000000000007e01000000000000800100000000000082010000000000008401000000000000860100000000000088010000000000008a010000000000008c010000000000008e01000000000000900100000000000092010000000000009401000000000000960100000000000098010000000000009a010000000000009c010000000000009e01000000000000a001000000000000a201000000000000a401000000000000a601000000000000a801000000000000aa01000000000000ac01000000000000ae01000000000000b001000000000000b201000000000000b401000000000000b601000000000000b801000000000000ba01000000000000bc01000000000000be01000000000000c001000000000000c201000000000000c401000000000000c601000000000000c801000000000000ca01000000000000cc01000000000000ce01000000000000d001000000000000d201000000000000d401000000000000d601000000000000d801000000000000da01000000000000dc01000000000000de01000000000000e001000000000000e201000000000000e401000000000000e601000000000000e801000000000000ea01000000000000ec01000000000000ee01000000000000f001000000000000f201000000000000f401000000000000f601000000000000f801000000000000fa01000000000000fc01000000000000fe01000000000000000200000000000002020000000000000402000000000000060200000000000008020000000000000a020000000000000c020000000000000e02000000000000100200000000000012020000000000001402000000000000160200000000000018020000000000001a020000000000001c020000000000001e02000000000000200200000000000022020000000000002402000000000000260200000000000028020000000000002a020000000000002c020000000000002e02000000000000300200000000000032020000000000003402000000000000360200000000000038020000000000003a020000000000003c020000000000003e02000000000000400200000000000042020000000000004402000000000000460200000000000048020000000000004a020000000000004c020000000000004e02000000000000500200000000000052020000000000005402000000000000560200000000000058020000000000005a020000000000005c020000000000005e02000000000000600200000000000062020000000000006402000000000000660200000000000068020000000000006a020000000000006c020000000000006e02000000000000700200000000000072020000000000007402000000000000760200000000000078020000000000007a020000000000007c020000000000007e02000000000000800200000000000082020000000000008402000000000000860200000000000088020000000000008a020000000000008c020000000000008e02000000000000900200000000000092020000000000009402000000000000960200000000000098020000000000009a020000000000009c020000000000009e02000000000000a002000000000000a202000000000000a402000000000000a602000000000000a802000000000000aa02000000000000ac02000000000000ae02000000000000b002000000000000b202000000000000b402000000000000b602000000000000b802000000000000ba02000000000000bc02000000000000be02000000000000c002000000000000c202000000000000c402000000000000c602000000000000c802000000000000ca02000000000000cc02000000000000ce02000000000000d002000000000000d202000000000000d402000000000000d602000000000000d802000000000000da02000000000000dc02000000000000de02000000000000e002000000000000e202000000000000e402000000000000e602000000000000e802000000000000ea02000000000000ec02000000000000ee02000000000000f002000000000000f202000000000000f402000000000000f602000000000000f802000000000000fa02000000000000fc02000000000000fe02000000000000000300000000000002030000000000000403000000000000060300000000000008030000000000000a030000000000000c030000000000000e03000000000000100300000000000012030000000000001403000000000000160300000000000018030000000000001a030000000000001c030000000000001e03000000000000200300000000000022030000000000002403000000000000260300000000000028030000000000002a030000000000002c030000000000002e03000000000000300300000000000032030000000000003403000000000000360300000000000038030000000000003a030000000000003c030000000000003e03000000000000400300000000000042030000000000004403000000000000460300000000000048030000000000004a030000000000004c030000000000004e03000000000000500300000000000052030000000000005403000000000000560300000000000058030000000000005a030000000000005c030000000000005e03000000000000600300000000000062030000000000006403000000000000660300000000000068030000000000006a030000000000006c030000000000006e03000000000000700300000000000072030000000000007403000000000000760300000000000078030000000000007a030000000000007c030000000000007e03000000000000800300000000000082030000000000008403000000000000860300000000000088030000000000008a030000000000008c030000000000008e03000000000000900300000000000092030000000000009403000000000000960300000000000098030000000000009a030000000000009c030000000000009e03000000000000a003000000000000a203000000000000a403000000000000a603000000000000a803000000000000aa03000000000000ac03000000000000ae03000000000000b003000000000000b203000000000000b403000000000000b603000000000000b803000000000000ba03000000000000bc03000000000000be03000000000000c003000000000000c203000000000000c403000000000000c603000000000000c803000000000000ca03000000000000cc03000000000000ce03000000000000d003000000000000d203000000000000d403000000000000d603000000000000d803000000000000da03000000000000dc03000000000000de03000000000000e003000000000000e203000000000000e403000000000000e603000000000000e803000000000000ea03000000000000ec03000000000000ee03000000000000f003000000000000f203000000000000f403000000000000f603000000000000f803000000000000fa03000000000000fc03000000000000fe03000000000000\"\nCameraAttributes::LUTControl::LUTSelector = \"Luminance\"\nCameraAttributes::DigitalIOControl::LineSelector = \"Line1\"\nCameraAttributes::DigitalIOControl::LineMode = \"Input\"\nCameraAttributes::DigitalIOControl::LineSelector = \"Line2\"\nCameraAttributes::DigitalIOControl::LineMode = \"Output\"\nCameraAttributes::DigitalIOControl::LineSelector = \"Line3\"\nCameraAttributes::DigitalIOControl::LineMode = \"Input\"\nCameraAttributes::DigitalIOControl::LineSelector = \"Line4\"\nCameraAttributes::DigitalIOControl::LineMode = \"Input\"\nCameraAttributes::DigitalIOControl::LineSelector = \"Line1\"\nCameraAttributes::DigitalIOControl::LineSelector = \"Line2\"\nCameraAttributes::DigitalIOControl::LineSource = \"UserOutput1\"\nCameraAttributes::DigitalIOControl::LineSelector = \"Line1\"\nCameraAttributes::DigitalIOControl::LineSelector = \"Line1\"\nCameraAttributes::DigitalIOControl::LineInverter = \"0\"\nCameraAttributes::DigitalIOControl::LineSelector = \"Line2\"\nCameraAttributes::DigitalIOControl::LineInverter = \"0\"\nCameraAttributes::DigitalIOControl::LineSelector = \"Line3\"\nCameraAttributes::DigitalIOControl::LineInverter = \"0\"\nCameraAttributes::DigitalIOControl::LineSelector = \"Line4\"\nCameraAttributes::DigitalIOControl::LineInverter = \"0\"\nCameraAttributes::DigitalIOControl::LineSelector = \"Line1\"\nCameraAttributes::DigitalIOControl::LineSelector = \"Line1\"\nCameraAttributes::DigitalIOControl::LineDebouncerTime = \"0.00000\"\nCameraAttributes::DigitalIOControl::LineSelector = \"Line3\"\nCameraAttributes::DigitalIOControl::LineDebouncerTime = \"0.00000\"\nCameraAttributes::DigitalIOControl::LineSelector = \"Line4\"\nCameraAttributes::DigitalIOControl::LineDebouncerTime = \"0.00000\"\nCameraAttributes::DigitalIOControl::LineSelector = \"Line1\"\nCameraAttributes::DigitalIOControl::LineSelector = \"Line2\"\nCameraAttributes::DigitalIOControl::LineMinimumOutputPulseWidth = \"0.000\"\nCameraAttributes::DigitalIOControl::LineSelector = \"Line1\"\nCameraAttributes::DigitalIOControl::UserOutputValueAll = \"0\"\nCameraAttributes::BslLightControl::BslLightControlMode = \"Off\"\nCameraAttributes::CounterAndTimerControl::TimerSelector = \"Timer1\"\nCameraAttributes::CounterAndTimerControl::TimerDuration = \"0.0\"\nCameraAttributes::CounterAndTimerControl::TimerSelector = \"Timer1\"\nCameraAttributes::CounterAndTimerControl::TimerSelector = \"Timer1\"\nCameraAttributes::CounterAndTimerControl::TimerDelay = \"0.0\"\nCameraAttributes::CounterAndTimerControl::TimerSelector = \"Timer1\"\nCameraAttributes::CounterAndTimerControl::TimerSelector = \"Timer1\"\nCameraAttributes::CounterAndTimerControl::TimerTriggerSource = \"ExposureStart\"\nCameraAttributes::CounterAndTimerControl::TimerSelector = \"Timer1\"\nCameraAttributes::CounterAndTimerControl::CounterSelector = \"Counter1\"\nCameraAttributes::CounterAndTimerControl::CounterEventSource = \"FrameStart\"\nCameraAttributes::CounterAndTimerControl::CounterSelector = \"Counter2\"\nCameraAttributes::CounterAndTimerControl::CounterEventSource = \"FrameStart\"\nCameraAttributes::CounterAndTimerControl::CounterSelector = \"Counter1\"\nCameraAttributes::CounterAndTimerControl::CounterSelector = \"Counter1\"\nCameraAttributes::CounterAndTimerControl::CounterResetSource = \"Off\"\nCameraAttributes::CounterAndTimerControl::CounterSelector = \"Counter2\"\nCameraAttributes::CounterAndTimerControl::CounterResetSource = \"Counter2End\"\nCameraAttributes::CounterAndTimerControl::CounterSelector = \"Counter1\"\nCameraAttributes::BslLightControl::BslLightControlTriggerMode = \"ExposureActive\"\nCameraAttributes::EventControl::EventSelector = \"ExposureEnd\"\nCameraAttributes::EventControl::EventNotification = \"Off\"\nCameraAttributes::EventControl::EventSelector = \"FrameStart\"\nCameraAttributes::EventControl::EventNotification = \"Off\"\nCameraAttributes::EventControl::EventSelector = \"FrameBurstStart\"\nCameraAttributes::EventControl::EventNotification = \"Off\"\nCameraAttributes::EventControl::EventSelector = \"FrameStartOvertrigger\"\nCameraAttributes::EventControl::EventNotification = \"Off\"\nCameraAttributes::EventControl::EventSelector = \"FrameBurstStartOvertrigger\"\nCameraAttributes::EventControl::EventNotification = \"Off\"\nCameraAttributes::EventControl::EventSelector = \"CriticalTemperature\"\nCameraAttributes::EventControl::EventNotification = \"Off\"\nCameraAttributes::EventControl::EventSelector = \"OverTemperature\"\nCameraAttributes::EventControl::EventNotification = \"Off\"\nCameraAttributes::EventControl::EventSelector = \"FrameStartWait\"\nCameraAttributes::EventControl::EventNotification = \"Off\"\nCameraAttributes::EventControl::EventSelector = \"FrameBurstStartWait\"\nCameraAttributes::EventControl::EventNotification = \"Off\"\nCameraAttributes::EventControl::EventSelector = \"ExposureEnd\"\nCameraAttributes::UserDefinedValueControl::UserDefinedValueSelector = \"Value1\"\nCameraAttributes::UserDefinedValueControl::UserDefinedValue = \"0\"\nCameraAttributes::UserDefinedValueControl::UserDefinedValueSelector = \"Value2\"\nCameraAttributes::UserDefinedValueControl::UserDefinedValue = \"0\"\nCameraAttributes::UserDefinedValueControl::UserDefinedValueSelector = \"Value3\"\nCameraAttributes::UserDefinedValueControl::UserDefinedValue = \"0\"\nCameraAttributes::UserDefinedValueControl::UserDefinedValueSelector = \"Value4\"\nCameraAttributes::UserDefinedValueControl::UserDefinedValue = \"0\"\nCameraAttributes::UserDefinedValueControl::UserDefinedValueSelector = \"Value5\"\nCameraAttributes::UserDefinedValueControl::UserDefinedValue = \"0\"\nCameraAttributes::UserDefinedValueControl::UserDefinedValueSelector = \"Value1\"\n"  # Attributes
      w123 = "cam1"  # Interface Name
      n66 = call <vilib>:"IMAQdx Open Camera.vi"("error in"="error in 2", "Session In"=w123) -> ("error out"=w121:errorcluster, "Session Out"=w122:T8)  [unwired: 1 in, 7 out]
      n67 = call <vilib>:"IMAQdx Read Attributes From String.vi"("error in"=w121, "Attributes String In"=w118, "Session In"=w122) -> ("error out"=w119:errorcluster, "Session Out"=w120:T8)  [unwired: 7 out]
      n68 = call <vilib>:"IMAQdx Configure Grab.vi"("error in"=w119, "Session In"=w120) -> ("error out"=w116:errorcluster, "Session Out"=w117:T8)  [unwired: 1 in, 7 out]
    }
    frame True {
    }
  }
  n69 = flat-sequence {
    tunnel: [w125] -> w4
    frame #0 {
      w125 = FALSE ("receive")
      n70 = local write "stop 2"(w125) -> ()
      n71 = local write "stop acq"(w125) -> ()
      n72 = local write "rec start"(w125) -> ()
      n73 = global write "Global 1.vi" "rec ready 2"(w125) -> ()
      n74 = global write "Global 1.vi" "rec ready"(w125) -> ()
    }
  }
  n75 = call "tm_initialize_40.vi"() -> ("error out"=w36:errorcluster, "Number Of Cameras"=w35:u32)  [unwired: 8 in, 2 out]
  n76 = Obtain Queue(name (unnamed)="test", element data type=u16[][] []) -> (queue out=w21:refnum<queue>, error out=w19:errorcluster)  [unwired: 3 in, 1 out]
  n77 = Obtain Queue(name (unnamed)="timestamp", element data type=0.0) -> (queue out=w20:refnum<queue>, error out=w18:errorcluster)  [unwired: 3 in, 1 out]
  n78 = Not Equal To 0?(x=w35) -> (x != 0?=w37:bool)
  n79 = case shown="True" w37 {
    tunnel: [w126 w205] -> w15
    tunnel: w36 -> [w126 w208]
    tunnel: w21 -> [_ w177]
    tunnel: w19 -> [_ w176]
    tunnel: w20 -> [_ w175]
    tunnel: w18 -> [_ w174]
    tunnel: w23 -> [_ _]
    tunnel: [_ w135] -> w13
    tunnel: [_ w134] -> w14
    tunnel: w11 -> [_ w133]
    tunnel: w9 -> [_ w130]
    tunnel: w4 -> [_ _]
    frame False {
    }
    frame True {
      w132 = 3  # Border Size
      w131 = "Basler monitor"  # Image Name
      w127 = FALSE
      w148 = u32 1852592 items=["SENSOR MODE"=4212128, "READOUT SPEED"=4211872, "READOUT DIRECTION"=4211904, "TRIGGER GLOBAL EXPOSURE"=2049680, "TRIGGER DELAY"=1066480, "INTERNAL TRIGGER HANDLING"=1066496, "SYNC READOUT SYSTEM BLANK"=1066528, "SENSOR TEMPERATURE"=2115232, "SENSOR COOLER STATUS"=2115280, "EXPOSURE TIME"=2049184, "DEFECT CORRECT MODE"=4670368, "BINNING"=4215968, "INTERNAL LINE SPEED"=4226000, "INTERNAL LINE INTERVAL"=4226016, "NUMBER OF OUTPUT TRIGGER CONNECTOR"=1852320, "OUTPUT TRIGGER SOURCE[0]"=1852576, "OUTPUT TRIGGER SOURCE[1]"=1852832, "OUTPUT TRIGGER SOURCE[2]"=1853088, "OUTPUT TRIGGER POLARITY[0]"=1852592, "OUTPUT TRIGGER POLARITY[1]"=1852848, "OUTPUT TRIGGER POLARITY[2]"=1853104, "OUTPUT TRIGGER ACTIVE[0]"=1852608, "OUTPUT TRIGGER ACTIVE[1]"=1852864, "OUTPUT TRIGGER ACTIVE[2]"=1853120, "OUTPUT TRIGGER DELAY[0]"=1852624, "OUTPUT TRIGGER DELAY[1]"=1852880, "OUTPUT TRIGGER DELAY[2]"=1853136, "OUTPUT TRIGGER PERIOD[0]"=1852640, "OUTPUT TRIGGER PERIOD[1]"=1852896, "OUTPUT TRIGGER PERIOD[2]"=1853152, "OUTPUT TRIGGER KIND[0]"=1852656, "OUTPUT TRIGGER KIND[1]"=1852912, "OUTPUT TRIGGER KIND[2]"=1853168, "OUTPUT TRIGGER BASE SENSOR[0]"=1852672, "OUTPUT TRIGGER BASE SENSOR[1]"=1852928, "OUTPUT TRIGGER BASE SENSOR[2]"=1853184, "OUTPUT TRIGGER PRE HSYNC COUNT"=1852704] ("Parameter")
      w159 = u32 2049680 items=["SENSOR MODE"=4212128, "READOUT SPEED"=4211872, "READOUT DIRECTION"=4211904, "TRIGGER GLOBAL EXPOSURE"=2049680, "TRIGGER DELAY"=1066480, "INTERNAL TRIGGER HANDLING"=1066496, "SYNC READOUT SYSTEM BLANK"=1066528, "SENSOR TEMPERATURE"=2115232, "SENSOR COOLER STATUS"=2115280, "EXPOSURE TIME"=2049184, "DEFECT CORRECT MODE"=4670368, "BINNING"=4215968, "INTERNAL LINE SPEED"=4226000, "INTERNAL LINE INTERVAL"=4226016, "NUMBER OF OUTPUT TRIGGER CONNECTOR"=1852320, "OUTPUT TRIGGER SOURCE[0]"=1852576, "OUTPUT TRIGGER SOURCE[1]"=1852832, "OUTPUT TRIGGER SOURCE[2]"=1853088, "OUTPUT TRIGGER POLARITY[0]"=1852592, "OUTPUT TRIGGER POLARITY[1]"=1852848, "OUTPUT TRIGGER POLARITY[2]"=1853104, "OUTPUT TRIGGER ACTIVE[0]"=1852608, "OUTPUT TRIGGER ACTIVE[1]"=1852864, "OUTPUT TRIGGER ACTIVE[2]"=1853120, "OUTPUT TRIGGER DELAY[0]"=1852624, "OUTPUT TRIGGER DELAY[1]"=1852880, "OUTPUT TRIGGER DELAY[2]"=1853136, "OUTPUT TRIGGER PERIOD[0]"=1852640, "OUTPUT TRIGGER PERIOD[1]"=1852896, "OUTPUT TRIGGER PERIOD[2]"=1853152, "OUTPUT TRIGGER KIND[0]"=1852656, "OUTPUT TRIGGER KIND[1]"=1852912, "OUTPUT TRIGGER KIND[2]"=1853168, "OUTPUT TRIGGER BASE SENSOR[0]"=1852672, "OUTPUT TRIGGER BASE SENSOR[1]"=1852928, "OUTPUT TRIGGER BASE SENSOR[2]"=1853184, "OUTPUT TRIGGER PRE HSYNC COUNT"=1852704] ("Parameter")
      w162 = u32 1852656 items=["SENSOR MODE"=4212128, "READOUT SPEED"=4211872, "READOUT DIRECTION"=4211904, "TRIGGER GLOBAL EXPOSURE"=2049680, "TRIGGER DELAY"=1066480, "INTERNAL TRIGGER HANDLING"=1066496, "SYNC READOUT SYSTEM BLANK"=1066528, "SENSOR TEMPERATURE"=2115232, "SENSOR COOLER STATUS"=2115280, "EXPOSURE TIME"=2049184, "DEFECT CORRECT MODE"=4670368, "BINNING"=4215968, "INTERNAL LINE SPEED"=4226000, "INTERNAL LINE INTERVAL"=4226016, "NUMBER OF OUTPUT TRIGGER CONNECTOR"=1852320, "OUTPUT TRIGGER SOURCE[0]"=1852576, "OUTPUT TRIGGER SOURCE[1]"=1852832, "OUTPUT TRIGGER SOURCE[2]"=1853088, "OUTPUT TRIGGER POLARITY[0]"=1852592, "OUTPUT TRIGGER POLARITY[1]"=1852848, "OUTPUT TRIGGER POLARITY[2]"=1853104, "OUTPUT TRIGGER ACTIVE[0]"=1852608, "OUTPUT TRIGGER ACTIVE[1]"=1852864, "OUTPUT TRIGGER ACTIVE[2]"=1853120, "OUTPUT TRIGGER DELAY[0]"=1852624, "OUTPUT TRIGGER DELAY[1]"=1852880, "OUTPUT TRIGGER DELAY[2]"=1853136, "OUTPUT TRIGGER PERIOD[0]"=1852640, "OUTPUT TRIGGER PERIOD[1]"=1852896, "OUTPUT TRIGGER PERIOD[2]"=1853152, "OUTPUT TRIGGER KIND[0]"=1852656, "OUTPUT TRIGGER KIND[1]"=1852912, "OUTPUT TRIGGER KIND[2]"=1853168, "OUTPUT TRIGGER BASE SENSOR[0]"=1852672, "OUTPUT TRIGGER BASE SENSOR[1]"=1852928, "OUTPUT TRIGGER BASE SENSOR[2]"=1853184, "OUTPUT TRIGGER PRE HSYNC COUNT"=1852704] ("Parameter")
      w172 = 2 items=["Internal"=1, "External"=2, "Software"=3, "Master Pulse"=4] ("Source")
      w173 = u32 4212128 items=["SENSOR MODE"=4212128, "READOUT SPEED"=4211872, "READOUT DIRECTION"=4211904, "TRIGGER GLOBAL EXPOSURE"=2049680, "TRIGGER DELAY"=1066480, "INTERNAL TRIGGER HANDLING"=1066496, "SYNC READOUT SYSTEM BLANK"=1066528, "SENSOR TEMPERATURE"=2115232, "SENSOR COOLER STATUS"=2115280, "EXPOSURE TIME"=2049184, "DEFECT CORRECT MODE"=4670368, "BINNING"=4215968, "INTERNAL LINE SPEED"=4226000, "INTERNAL LINE INTERVAL"=4226016, "NUMBER OF OUTPUT TRIGGER CONNECTOR"=1852320, "OUTPUT TRIGGER SOURCE[0]"=1852576, "OUTPUT TRIGGER SOURCE[1]"=1852832, "OUTPUT TRIGGER SOURCE[2]"=1853088, "OUTPUT TRIGGER POLARITY[0]"=1852592, "OUTPUT TRIGGER POLARITY[1]"=1852848, "OUTPUT TRIGGER POLARITY[2]"=1853104, "OUTPUT TRIGGER ACTIVE[0]"=1852608, "OUTPUT TRIGGER ACTIVE[1]"=1852864, "OUTPUT TRIGGER ACTIVE[2]"=1853120, "OUTPUT TRIGGER DELAY[0]"=1852624, "OUTPUT TRIGGER DELAY[1]"=1852880, "OUTPUT TRIGGER DELAY[2]"=1853136, "OUTPUT TRIGGER PERIOD[0]"=1852640, "OUTPUT TRIGGER PERIOD[1]"=1852896, "OUTPUT TRIGGER PERIOD[2]"=1853152, "OUTPUT TRIGGER KIND[0]"=1852656, "OUTPUT TRIGGER KIND[1]"=1852912, "OUTPUT TRIGGER KIND[2]"=1853168, "OUTPUT TRIGGER BASE SENSOR[0]"=1852672, "OUTPUT TRIGGER BASE SENSOR[1]"=1852928, "OUTPUT TRIGGER BASE SENSOR[2]"=1853184, "OUTPUT TRIGGER PRE HSYNC COUNT"=1852704] ("Parameter")
      w128 = 0 ("Frame Count")
      w178 = u32 2049184 items=["SENSOR MODE"=4212128, "CCD MODE"=4212384, "READOUT MODE"=4211872, "ACTIVE VIEW INDEX"=4343136, "BITS PER CHANNEL"=4342976, "IMAGE PIXEL TYPE"=4343296, "BINNING"=4215968, "EXPOSURE TIME"=2049184, "CONTRAST GAIN"=3163312, "CONTRAST OFFSET"=3163328, "LIGHT MODE"=2114720, "SENSITIVITY"=2114992, "PHOTON IMAGING MODE"=2115200, "HIGH DYNAMIC RANGE MODE"=3163360, "WHITE BALANCE"=3163568, "TEMPERATURE"=2115232, "TEMPERATURE TARGET"=2115264, "SENSOR COOLER FAN"=2115296, "LINEBUNDLE HEIGHT"=4212192, "MECHANICAL SHUTTER"=2115488, "BACK FOCUS POSITION"=8422304, "TRIGGER CONNECTOR"=1066432, "TRIGGER SOURCE"=1066144, "OUTPUT TRIGGER SOURCE"=1852576, "TRIGGER GLOBAL EXPOSURE"=2049680, "FIRST TRIGGER BEHAVIOR"=2049696, "CHANNEL SYNC"=1852352, "READOUT DIRECTION"=4211904, "PRE HSYNC COUNT"=1852704] ("Parameter")
      w179 = u32 4211872 items=["SENSOR MODE"=4212128, "CCD MODE"=4212384, "READOUT MODE"=4211872, "ACTIVE VIEW INDEX"=4343136, "BITS PER CHANNEL"=4342976, "IMAGE PIXEL TYPE"=4343296, "BINNING"=4215968, "EXPOSURE TIME"=2049184, "CONTRAST GAIN"=3163312, "CONTRAST OFFSET"=3163328, "LIGHT MODE"=2114720, "SENSITIVITY"=2114992, "PHOTON IMAGING MODE"=2115200, "HIGH DYNAMIC RANGE MODE"=3163360, "WHITE BALANCE"=3163568, "TEMPERATURE"=2115232, "TEMPERATURE TARGET"=2115264, "SENSOR COOLER FAN"=2115296, "LINEBUNDLE HEIGHT"=4212192, "MECHANICAL SHUTTER"=2115488, "BACK FOCUS POSITION"=8422304, "TRIGGER CONNECTOR"=1066432, "TRIGGER SOURCE"=1066144, "OUTPUT TRIGGER SOURCE"=1852576, "TRIGGER GLOBAL EXPOSURE"=2049680, "FIRST TRIGGER BEHAVIOR"=2049696, "CHANNEL SYNC"=1852352, "READOUT DIRECTION"=4211904, "PRE HSYNC COUNT"=1852704] ("Parameter")
      w204 = 1 items=["Snap", "Sequence"] ("Capture mode")
      n80 = call "tm_opencamera_40.vi"("error in (no error)"=w208, "Camera Index"=u32 0) -> ("error out"=w181:errorcluster, "Handle out"=w180:u32)  [unwired: 7 in, 1 out]
      n81 = call "tm_setparameter_40.vi"("error in (no error)"=w181, "Value in"=3.0 ("Scan Mode"), "Parameter"=w179, "Handle in"=w180) -> ("error out"=w182:errorcluster, "Handle out"=w183:u32)  [unwired: 6 in]
      n82 = call "tm_setparameter_40.vi"("error in (no error)"=w182, "Value in"="Exposure", "Parameter"=w178, "Handle in"=w183) -> ("error out"=w156:errorcluster, "Handle out"=w158:u32)  [unwired: 6 in]
      n83 = call "tm_setparameter_40.vi"("error in (no error)"=w156, "Value in"=5.0, "Parameter"=w159, "Handle in"=w158) -> ("error out"=w155:errorcluster, "Handle out"=w157:u32)  [unwired: 6 in]
      n84 = Bundle("H Offset"=0, "V Offset"="V Offset", "H Width"=2304, "V Width"="V Width") -> (w186:T11)  [unwired: 1 in]
      n85 = call "tm_setarea_40.vi"("error in (no error)"=w155, "Sub Region"=w186, "Handle in"=w157) -> ("error out"=w170:errorcluster, "Handle out"=w171:u32)  [unwired: 7 in]
      n86 = call "tm_setparameter_40.vi"("error in (no error)"=w170, "Value in"=1.0, "Parameter"=w173, "Handle in"=w171) -> ("error out"=w168:errorcluster, "Handle out"=w169:u32)  [unwired: 6 in]
      n87 = call "tm_inputtriggersource_40.vi"("error in (no error)"=w168, "External Options"=cluster{"Polarity":i32, "Delay":dbl} {"Polarity"=2, "Delay"=0.0}, "Source"=w172, "Handle in"=w169) -> ("error out"=w166:errorcluster, "Handle out"=w167:u32)  [unwired: 6 in]
      n88 = call "tm_setoutputtrigger_40.vi"("error in (no error)"=w166, "Type"=cluster{"Mode":u32, "Polarity":u32} {"Mode"=2, "Polarity"=1}, "Handle in"=w167) -> ("error out"=w152:errorcluster, "Handle out"=w151:u32)  [unwired: 7 in]
      n89 = call "tm_setparameter_40.vi"("error in (no error)"=w152, "Value in"=2.0, "Parameter"=w148, "Handle in"=w151) -> ("error out"=w149:errorcluster, "Handle out"=w150:u32)  [unwired: 6 in]
      n90 = call "tm_setparameter_40.vi"("error in (no error)"=w149, "Value in"=2.0, "Parameter"=w162, "Handle in"=w150) -> ("error out"=w161:errorcluster, "Handle out"=w160:u32)  [unwired: 6 in]
      n91 = call "tm_getarea_40.vi"("error in (no error)"=w161, "Handle in"=w160) -> ("error out"=w199:errorcluster, "Sub Region"=w195:T13, "Handle out"=w198:u32)  [unwired: 7 in]
      n92 = Unbundle(w195) -> ("V Offset"=w197:cluster{"Value":i32, "Limits":T12}, "V Size"=w196:cluster{"Value":i32, "Limits":T12})  [unwired: 2 out]
      n93 = Unbundle By Name(w197) -> ("Value"=w192:i32, "Limits"=w191:T12)
      "SVO" <- w192
      n94 = Unbundle By Name(w196) -> ("Value"=w194:i32, "Limits"=w193:T12)
      "SVW" <- w194
      n95 = call "tm_preparecapture_40.vi"("error in (no error)"=w199, "Frames"="buffer frames", "Capture mode"=w204, "Handle in"=w198) -> ("error out"=w146:errorcluster, "Handle out"=w145:u32)  [unwired: 4 in, 2 out]
      n96 = call "tm_startcapture_40.vi"("error in (no error)"=w146, "Handle in"=w145) -> ("error out"=w141:errorcluster, "Handle out"=w143:u32)  [unwired: 8 in]
      n97 = property on="V Offset" class="DigNum (strict)"("Value"=w192, "Data Range"=w191) -> ()  [unwired: 2 in, 2 out]
      n98 = property on="V Width" class="DigNum (strict)"("Value"=w194, "Data Range"=w193) -> ()  [unwired: 2 in, 2 out]
      n99 = flat-sequence {
        tunnel: [w219] -> w144
        tunnel: w143 -> [w219]
        tunnel: [w218] -> w142
        tunnel: w141 -> [w218]
        frame #0 {
          n100 = local write "sCMOS"(TRUE ("Boolean")) -> ()
        }
      }
      n101 = call "IMAQ Create"("Border Size"=w132, "Image Name"=w131) -> ("New Image"=w129:T14)  [unwired: 2 in, 2 out]
      n102 = while {
        tunnel: w142 -> [w269]
        tunnel: [w268] -> w140
        tunnel: [w267] -> w139
        shift-right: [w241] -> _
        shift-left: w128 -> [w240]
        tunnel: w177 -> [w264]
        tunnel: w176 -> [w223]
        shift-right: [w263] -> _
        shift-left: w128 -> [w248]
        tunnel: w175 -> [w262]
        tunnel: w174 -> [w261]
        tunnel: "buffer frames" -> [w260]
        tunnel: w144 -> [w256]
        shift-right: [w252] -> _
        shift-left: w128 -> [w253]
        shift-right: [w220] -> _
        shift-left: w127 -> [w250]
        tunnel: [w246] -> w135
        tunnel: [w245] -> w134
        tunnel: w133 -> [w243]
        tunnel: w130 -> [w230]
        tunnel: w129 -> [w231]
        shift-right: [w228] -> _
        shift-left: w128 -> [w229]
        shift-right: [w225] -> _
        shift-left: w127 -> [w226]
        i -> [w258]
        stop <- w270 stop-if-true
        # "(slaveで) rec readyがONになったらバッファにたまった最後の"
        # "frame countが更新されたら読みだす"
        n103 = local read "REC"() -> (w225:bool)
        n104 = Not Equal?(x=w225, y=w226) -> (x != y?=w227:bool)
        n105 = case shown="True" w227 {
          frame False {
          }
          frame True {
            n106 = global write "Global 1.vi" "record"(TRUE) -> ()
          }
        }
        n107 = global read "Global 1.vi" "rec ready"() -> (w220:bool)
        "rec ready" <- w220
        n108 = local read "master(F)/slave(T)"() -> (w221:bool)
        n109 = call "tm_getcaptureinfo_40.vi"("error in (no error)"=w269, "Handle in"=w256) -> ("error out"=w265:errorcluster, "Frame Count"=w242:i32, "Frame Index"=w257:i32, "Handle out"=w266:u32)  [unwired: 6 in]
        "Frame Index" <- w257
        "Frame Count 2" <- w242
        n110 = Not Equal?(x=w220, y=w250) -> (x != y?=w224:bool)
        n111 = Subtract(x=w242, y=w240) -> (x-y=w222:i32)
        n112 = case shown="True" w224 {
          tunnel: w253 -> [w275 _]
          tunnel: [w275 w281] -> w252
          tunnel: w242 -> [_ w281]
          tunnel: w221 -> [_ w279]
          tunnel: "one PC" -> [_ w278]
          tunnel: w248 -> [w274 _]
          tunnel: [w274 0 ("Frame Count")] -> w247
          tunnel: w223 -> [_ w276]
          frame False {
          }
          frame True {
            n113 = flat-sequence {
              tunnel: w279 -> [w287]
              tunnel: w278 -> [w286]
              tunnel: w276 -> [w285]
              frame #0 {
                n114 = case shown="False" w287 {
                  tunnel: w286 -> [w289 _]
                  tunnel: w285 -> [w288 _]
                  frame False {
                    # "masterの動作"
                    n115 = flat-sequence {
                      tunnel: w289 -> [w301]
                      tunnel: w288 -> [_]
                      frame #0 {
                        n116 = call "datetimestring for folder name.vi"() -> ("concatenated string"=w299:string)  [unwired: 1 in]
                        n117 = Concatenate Strings(w299, "foldername header") -> (w296:string)
                        "folder name" <- w296
                        n118 = case shown="False" w301 {
                          tunnel: w296 -> [w302 _]
                          frame False {
                            n119 = local read "frames to record"() -> (w305:u32)
                            n120 = Bundle("frames to record"=w305, w302) -> (w304:cluster{"frames to record":u32, string})  [unwired: 1 in]
                            n121 = Flatten To String(anything=w304) -> (data string=w303:string)  [unwired: 3 in, 2 out]
                            n122 = while {
                              tunnel: w303 -> [w315]
                              stop <- w307 stop-if-true
                              w310 = 100  # timeout ms
                              n123 = call "UDPsender.vi"("receiver's port"="cam receive port", "sender's port"="cam send port", "timeout ms"=w310, "r-t"=TRUE, "Receiver's IP"="slave IP", "data in"=w315) -> ("error"=w309:bool, "r-t time [s]"=→"r-t time [s]":dbl)  [unwired: 4 in]
                              n124 = Not(x=w309) -> (.not. x?=w308:bool)
                              n125 = Or(x="force", y=w308) -> (x .or. y?=w307:bool)
                            }
                          }
                          frame True {
                          }
                        }
                        n126 = local read "frames to record"() -> (w297:u32)
                        n127 = global read "global for picoscope.vi" "g2 period [us]"() -> (w298:dbl)
                        n128 = Bundle("g2 period [us]"=w298, "frames to record"=w297, w296) -> (w294:T15)  [unwired: 1 in]
                        n129 = Flatten To String(anything=w294) -> (data string=w293:string)  [unwired: 3 in, 2 out]
                        n130 = call "UDPsender.vi"("receiver's port"="pico receive port", "sender's port"="pico send port", "r-t"=FALSE, "Receiver's IP"="picoscope  IP", "data in"=w293) -> ()  [unwired: 5 in, 2 out]
                      }
                      frame #1 {
                        n131 = global write "Global 1.vi" "rec ready 2"(TRUE) -> ()
                      }
                    }
                  }
                  frame True {
                  }
                }
              }
              frame #1 {
                "rec start" <- TRUE
              }
            }
            n132 = global write "Global 1.vi" "calib"("calib") -> ()
            n133 = case shown="True" "calib" {
              frame False {
              }
              frame True {
                n134 = call "Enable Output.vi"("Enable Output (T: Enable)"=FALSE, "VISA resource name"=refnum<visa-resource-name> "USB0::0x1AB1::0x0641::DG4E223801593::INSTR") -> ()  [unwired: 2 in, 8 out]
                n135 = global read "global for picoscope.vi" "frames for calib"() -> (w282:i32)
                n136 = local write "frames to record"(w282) -> ()
              }
            }
          }
        }
        n137 = global write "global for picoscope.vi" "calib/monitor"("calib/monitor") -> ()
        n138 = local read "REC"() -> (w235:bool)
        n139 = Compound Arithmetic op=AND(invert w235, "calib/monitor") -> (w234:bool)
        n140 = global read "global for picoscope.vi" "Nv"() -> (w237:i32)
        n141 = Select(t=w237, s=w234, f=1) -> (s? t:f=w238:i32)
        n142 = Greater Or Equal?(x=w222, y=w238) -> (x >= y?=w239:bool)
        n143 = case shown="True" w239 {
          tunnel: [w323 w355] -> w268
          tunnel: [w322 w354] -> w267
          tunnel: w266 -> [w323 w353]
          tunnel: w265 -> [w322 w352]
          tunnel: w257 -> [_ w351]
          tunnel: w264 -> [_ w350]
          tunnel: w223 -> [_ w349]
          tunnel: w247 -> [w321 w348]
          tunnel: [w321 w347] -> w263
          tunnel: w222 -> [_ w340]
          tunnel: w262 -> [_ w345]
          tunnel: w261 -> [_ w344]
          tunnel: w260 -> [_ w343]
          tunnel: "monitor" -> [_ w341]
          tunnel: [_ w338] -> w246
          tunnel: [_ w337] -> w245
          tunnel: w243 -> [_ w335]
          tunnel: w235 -> [_ w331]
          tunnel: w242 -> [_ w334]
          tunnel: [w320 w334] -> w241
          tunnel: w240 -> [w320 _]
          tunnel: "calib/monitor" -> [_ w333]
          tunnel: w231 -> [_ w330]
          tunnel: w230 -> [_ w329]
          tunnel: w229 -> [w319 w325]
          tunnel: [w319 w327] -> w228
          tunnel: w220 -> [_ w324]
          frame False {
          }
          frame True {
            n144 = Increment(x=w348) -> (x+1=w347:i32)
            n145 = In Range and Coerce(upper limit=w343, x=w340, lower limit=1) -> (coerced(x)=w328:i32)  [unwired: 1 out]
            n146 = for {
              N: w328 -> [w363]
              tunnel: w351 -> [w359]
              tunnel: [w369] -> w332 mode=indexing
              tunnel: w350 -> [w371]
              tunnel: w349 -> [w370]
              tunnel: w352 -> [w372]
              tunnel: [w374] -> w354
              tunnel: w353 -> [w373]
              tunnel: [w375] -> w355
              tunnel: w345 -> [w367]
              tunnel: w344 -> [w366]
              tunnel: w343 -> [w365]
              tunnel: w324 -> [w356]
              i -> [w361]
              # "read buffer of sCMOS"
              n147 = local read "REC"() -> (w357:bool)
              n148 = Compound Arithmetic op=ADD(invert w363, 1 ("value"), w361, w359) -> (w360:i32)
              n149 = Quotient & Remainder(x=w360, y=w365) -> (x-y*floor(x/y)=w368:i32)  [unwired: 1 out]
              n150 = And(x=w357, y=w356) -> (x .and. y?=w358:bool)
              n151 = call "tm_getframe16_40.vi"("error in (no error)"=w372, "Frame Index"=w368, "Handle in"=w373) -> ("error out"=w374:errorcluster, "Timestamp"=w364:dbl, "Data"=w369:u16[][], "Handle out"=w375:u32)  [unwired: 5 in]
              "Timestamp" <- w364
              n152 = case shown="False" w358 {
                tunnel: w371 -> [_ w394]
                tunnel: w370 -> [_ w393]
                tunnel: w369 -> [w379 w392]
                tunnel: w367 -> [_ w391]
                tunnel: w366 -> [_ w390]
                tunnel: w364 -> [w377 w389]
                frame False {
                  # "send image frames by UDP at monitor mode"
                  n153 = local read "master(F)/slave(T)"() -> (w376:bool)
                  n154 = case shown="False" w376 {
                    tunnel: w377 -> [w381 _]
                    frame False {
                      n155 = call "current time (HHMMSS.SSS-to-SSSSS.SSS).vi"() -> ("Numeric"=w382:dbl)  [unwired: 11 in]
                      n156 = Subtract(x=w382, y=w381) -> (x-y=→"time ofst":dbl)
                    }
                    frame True {
                    }
                  }
                  n157 = case shown="True" "UDP send at monitor" {
                    tunnel: w379 -> [_ w388]
                    tunnel: w377 -> [_ w383]
                    frame False {
                    }
                    frame True {
                      w386 = 65507  # Packet size
                      n158 = call "UDP volume send (subVI).vi"("timestamp"=w383, "Packet size"=w386, "local port"="img send port", "port of receiver"="img receive port", "address"="img process IP", "frame data"=w388) -> ()  [unwired: 5 in, 1 out]
                    }
                  }
                }
                frame True {
                  n159 = Enqueue Element(queue=w394, element=w392, error in (no error)=w393) -> ()  [unwired: 1 in, 3 out]
                  n160 = Enqueue Element(queue=w391, element=w389, error in (no error)=w390) -> ()  [unwired: 1 in, 3 out]
                }
              }
            }
            n161 = Add(x=w328, y=w325) -> (x+y=w326:i32)
            n162 = Select(t=w326, s=w324, f=w325) -> (s? t:f=w327:i32)
            n163 = local read "master(F)/slave(T)"() -> (w336:bool)
            n164 = Not(x=w331) -> (.not. x?=w339:bool)
            n165 = And(x=w341, y=w339) -> (x .and. y?=w342:bool)
            n166 = case shown="True" w342 {
              tunnel: w332 -> [_ w408]
              tunnel: [_ w425] -> w338
              tunnel: [_ w424] -> w337
              tunnel: w336 -> [_ w423]
              tunnel: w335 -> [_ w422]
              tunnel: w333 -> [_ w405]
              tunnel: w330 -> [_ w396]
              tunnel: w329 -> [_ w395]
              frame False {
              }
              frame True {
                n167 = case shown="False" w423 {
                  tunnel: [w469 _] -> w425
                  tunnel: [w450 _] -> w424
                  tunnel: w408 -> [w479 _]
                  tunnel: w422 -> [w477 _]
                  tunnel: w405 -> [w471 _]
                  tunnel: w396 -> [w452 _]
                  tunnel: w395 -> [w451 _]
                  frame False {
                    # "Bright Field image monitor"
                    n168 = call "set gain and exp time for Basler acA2500-60um (SubVI).vi"("Acquisition Control::Exposure Time"="BF Exp Time [us]", "Analog Control::Gain"="BF Gain", "Session Out"=w451, "Refnum in"=w452) -> ("Refnum out"=w450:T14)  [unwired: 6 in, 1 out]
                    n169 = call "IMAQ ImageToArray"("Image"=w450) -> ("error out"=w469:errorcluster, "Image Pixels (U8)"=w467:u8[][])  [unwired: 3 in, 3 out]
                    n170 = Array Size(array=w467) -> (size(s)=w462:i32[])
                    n171 = Subtract(x=1.0, y="ROI ratio [0-1]") -> (x-y=w465:dbl)
                    n172 = Divide(x=w465, y=2.0) -> (x/y=w463:dbl)
                    n173 = Multiply(x=w462, y=w463) -> (x*y=w459:dbl[])
                    n174 = Multiply(x=w462, y="ROI ratio [0-1]") -> (x*y=w460:dbl[])
                    n175 = Index Array(array=w459) -> (element #1=w456:dbl, element #2=w455:dbl)  [unwired: 2 in]
                    n176 = Index Array(array=w460) -> (element #1=w458:dbl, element #2=w457:dbl)  [unwired: 2 in]
                    n177 = Array Subset(array=w467, index (row)=w456, length (row)=w458, index (col)=w455, length (col)=w457) -> (w468:u8[][])
                    n178 = local read "overlay FL to BF"() -> (w478:bool)
                    n179 = case shown="True" w478 {
                      tunnel: w479 -> [_ w493]
                      tunnel: w468 -> [w487 w492]
                      tunnel: [w486 w491] -> w476
                      tunnel: w477 -> [_ w490]
                      tunnel: w471 -> [_ w488]
                      frame False {
                        n180 = Multiply(x=u8 0 ("Numerisch"), y=w487) -> (x*y=w486:u8[][])
                      }
                      frame True {
                        n181 = call "overlay oblique sliced FL imgs to BF img-2 (SubVI).vi"("calib(F)/monitor(T)"=w488, "config"="config", "scan pos in"=w490, "image in"=w493, "BF image in"=w492) -> ("overlaid image"=w491:u16[][])  [unwired: 2 in]
                      }
                    }
                    n182 = call "reverse imageU16.vi"("output array in"=w468, "reverse v"=FALSE, "reverse h"=FALSE) -> ("output array out"=w474:u16[][])
                    n183 = call "reverse imageU16.vi"("output array in"=w476, "reverse v"=TRUE) -> ("output array out"=w475:u16[][])  [unwired: 1 in]
                    n184 = Build Array(w474, w475) -> (w481:u16[][][])
                    n185 = control-ref of="BF"() -> (w483:refnum<vi>)
                    n186 = call "create multi-color image U16(SubVI).vi"("Zoom"="Zoom", "Array"=w481, "Cluster"="color scale", "Picture in"=w483) -> ("new picture 2"=→"BF":picture)  [unwired: 7 in]
                  }
                  frame True {
                  }
                }
                n187 = Boolean To (0,1)(Boolean=w405) -> (0, 1=w404:i16)
                n188 = Multiply(x=w404, y="page") -> (x*y=w402:i32)
                n189 = Index Array(array=w408, index (dim 0)=w402) -> (element=w409:u16[][])  [unwired: 2 in]
                n190 = control-ref of="Image"() -> (w427:refnum<vi>)
                n191 = call "Color config for intensity map U16 (SubVI).vi"("IntensityGraph ref in"=w427, "max adjust"="max adjust", "color"="color 2", "image in"=w409) -> ("max value"=→"max value":u16, "image out"=w400:u16[][])  [unwired: 5 in, 1 out]
                n192 = Transpose 2D Array(2D array=w400) -> (transposed array=w407:u16[][])
                n193 = case shown="True" "avg" {
                  tunnel: [w429 w436] -> w401
                  tunnel: w400 -> [w429 w434]
                  tunnel: 0 -> [_ w431]
                  tunnel: u32 0 -> [_ w430]
                  frame False {
                  }
                  frame True {
                    n194 = To Unsigned Long Integer(number=w434) -> (unsigned 32bit integer=w433:u32[][])
                    n195 = Multiply(x=w433, y=w430) -> (x*y=w435:u32[][])
                    n196 = feedback #1(w431) -> (w440:i32)
                    n197 = Increment(x=w440) -> (x+1=w439:i32)
                    n198 = feedback-in #1(w439) -> ()
                    n199 = feedback #2(w435) -> (w441:u32[][])
                    n200 = Add(x=w433, y=w441) -> (x+y=w432:u32[][])
                    n201 = feedback-in #2(w432) -> ()
                    n202 = Reciprocal(x=w439) -> (1/x=w438:dbl)
                    n203 = Multiply(x=w432, y=w438) -> (x*y=w437:dbl[][])
                    n204 = To Unsigned Word Integer(number=w437) -> (unsigned 16bit integer=w436:u16[][])
                  }
                }
                "Image" <- w401
                n205 = for {
                  tunnel: w407 -> [w443] mode=indexing
                  tunnel: [w442] -> w406 mode=indexing
                  n206 = To Unsigned Long Integer(number=w443) -> (unsigned 32bit integer=w444:u32[])
                  n207 = Add Array Elements(numeric array=w444) -> (sum=w442:u32)
                }
                "img projection on x" <- w406
                n208 = local read "config"() -> (w415:T2)
                n209 = Unbundle By Name(w415) -> ("AOD scan speed ratio"=w413:dbl, "Nx"=w414:dbl)
                n210 = local read "frame's init pos in x"() -> (w411:dbl[][])
                n211 = Bundle By Name(cluster=T10 {"xy cut pos correct"=[[0.0, 0.0, 0.0, -7.0], [0.0, 0.0, 0.0, -7.0], [0.0, 0.0, 0.0, -7.0], [0.0, 0.0, 0.0, -7.0], [0.0, 0.0, 0.0, -7.0], [0.0, 0.0, 0.0, 0.0], [0.0, 0.0, 0.0, 0.0], [0.0, 0.0, 0.0, 0.0], [0.0, 0.0, 0.0, 0.0], [0.0, 0.0, 0.0, 0.0]], "3D reconst config"={"xyz pos"=[271, 288, 150], "color 4"={"color array"=[0, 8388736, 16711680, 16776960, 16776960, 16711680, 16448250, 16448250], "num of colors"=4, "max"=7000.900000000023, "min"=100.0}, "autogain"=TRUE, "zoom"=1.0, "slice(T)/stack(F)"=FALSE, "xy cut mag"=1.0000000000000004, "xy cut ofst"=0.0, "z/xy comp"=0.9999999999999998, "y shift comp"=0.0, "max plot"=TRUE, "oblique angle [deg]"=45.0, "voxel size z [um]"=5.066639031844781, "voxel size xy[um]"=0.455, "reverse v"=FALSE, "reverse h"=TRUE, "3D reconstruction"=TRUE, "reverse z"=FALSE}, "xy cut pos"=[[0.0, 4.540011367701254, 4.853687897950067, 5.137490472936861], [207.4696403005795, 211.47606963402166, 212.00384284364657, 211.78310750754565], [421.4617608333166, 425.35948216288944, 425.8192091410847, 426.1901440855853], [642.40206546069, 646.4425179098467, 646.8897974066831, 647.0541041606228], [871.5767939231397, 875.391532043652, 875.6172463722967, 876.1035279773913], [1108.4465553617717, 1112.4031947697777, 1112.9766087443859, 1112.9317978114932], [1350.135151750549, 1354.1980096661523, 1354.7506778384952, 1354.8104257490188], [1587.7666990483574, 1591.187266925832, 1591.5457543889736, 1591.7075716466416], [1812.700155695724, 1816.1970681255343, 1816.7497362978775, 1816.9289800294482], [2008.714793817587, 2011.9801830941183, 2012.2158554078503, 2013.1535656702342]], "AOD scan speed ratio"=5.0, "Nx"=224.4, "stack method"=enum."0pad to z", "y shift"=-6} ("config in"), "stack method"=T9."none", "3D reconst config"="3D config", "xy cut pos correct"="xy cut pos correct", "y shift"=0, "AOD scan speed ratio"=w413, "Nx"=w414, "xy cut pos"=w411) -> (w420:T10)
                n212 = case shown="True" FALSE {
                  tunnel: w420 -> [_ w449]
                  tunnel: w408 -> [_ w448]
                  frame False {
                  }
                  frame True {
                    n213 = local read "cropcalib ch2"() -> (→"cropcalib ch2 2":dbl[][][])
                    n214 = local read "cropcalib ch1"() -> (w446:dbl[][][])
                    n215 = local read "cropcalib"() -> (w447:bool)
                    n216 = call "reconstruct 3D oblique image without config-2 (SubVI).vi"("image in"=w448, "config in"=w449, "cropcalib"=w447, "cropcalib data"=w446) -> ()  [unwired: 4 in, 8 out]
                  }
                }
              }
            }
            "buffers to read" <- w340
          }
        }
        "Frame Count" <- w263
        n217 = Subtract(x=w242, y=w252) -> (x-y=→"x-y":i32)
        n218 = local read "REC"() -> (w255:bool)
        n219 = Unbundle By Name(w267) -> ("status"=w271:bool)
        n220 = Greater Or Equal?(x=w228, y="frames to record") -> (x >= y?=w254:bool)
        n221 = global write "global for picoscope.vi" "frames to record"("frames to record") -> ()
        n222 = And(x=w254, y=w255) -> (x .and. y?=w244:bool)
        n223 = global write "Global 1.vi" "rec stop [Cam->Pico]"(w244) -> ()
        n224 = Compound Arithmetic op=OR(w244, w271, "stop") -> (w270:bool)
        "result" <- w270
        "Numeric" <- w258
        "stop 2" <- "stop"
      }
      n225 = flat-sequence {
        tunnel: [w216] -> w137
        tunnel: w140 -> [w216]
        tunnel: [w215] -> w138
        tunnel: w139 -> [w215]
        frame #0 {
          n226 = local read "pico receive port"() -> (w209:u16)
          n227 = local read "pico send port"() -> (w210:u16)
          n228 = local read "picoscope  IP"() -> (w211:string)
          n229 = local write "sCMOS"(FALSE ("Boolean")) -> ()
          n230 = call "UDPsender.vi"("receiver's port"=w209, "sender's port"=w210, "r-t"=FALSE, "Receiver's IP"=w211, "data in"="a") -> ()  [unwired: 5 in, 2 out]
        }
      }
      n231 = call "tm_stopcapture_40.vi"("error in (no error)"=w138, "Handle in"=w137) -> ("error out"=w201:errorcluster, "Handle out"=w202:u32)  [unwired: 8 in]
      n232 = call "tm_unpreparecapture_40.vi"("error in (no error)"=w201, "Handle in"=w202) -> ("error out"=w200:errorcluster, "Handle out"=w203:u32)  [unwired: 8 in]
      n233 = call "tm_closecamera_40.vi"("error in (no error)"=w200, "Handle in"=w203) -> ("error out"=w206:errorcluster)  [unwired: 9 in]
      n234 = call "tm_deinitialize_40.vi"("error in (no error)"=w206) -> ("error out"=w205:errorcluster)  [unwired: 10 in]
    }
  }
  "error out" <- w15
  n235 = while {
    tunnel: ["REC"] -> w30
    tunnel: w21 -> [w509]
    tunnel: w19 -> [w510]
    tunnel: w20 -> [w511]
    tunnel: [w508] -> w10
    tunnel: [w511] -> w27
    tunnel: [w510] -> w28
    tunnel: [w509] -> w29
    tunnel: w18 -> [w508]
    stop <- w507 stop-if-true
    # "記録しないかどうかはさいごまでわからないので、ここで保留にしておく。結局記録しない場合は手動でstop2がONになるので、これで終わる。"
    n236 = vi-ref "PicoScope4000aExampleStreaming without queue220623.vi"() -> (w500:refnum<vi>)
    n237 = property class="VI"(reference=w500) -> ("Exec.State"=w499:T16)  [unwired: 1 in, 2 out]
    n238 = local read "calib/monitor"() -> (w503:bool)
    n239 = Less?(x=w499, y=2) -> (x < y?=w496:bool)
    n240 = And(x="control picoscope dependent enable", y=w496) -> (x .and. y?=w495:bool)
    n241 = Or(x=w503, y=w495) -> (x .or. y?=w497:bool)
    n242 = Select(t=u8 2, s=w497, f=u8 0) -> (s? t:f=w504:u8)
    n243 = property on="REC" class="Bool (strict)"("DisabledEnum"=w504) -> ()  [unwired: 2 in, 2 out]
    n244 = local read "stop 2"() -> (w506:bool)
    n245 = Or(x="REC", y=w506) -> (x .or. y?=w507:bool)
  }
  n246 = case shown="True" "master(F)/slave(T)" {
    frame False {
    }
    frame True {
      n247 = flat-sequence {
        tunnel: [w515] -> w513
        tunnel: [w514] -> w512
        tunnel: w513 -> [w532]
        tunnel: w512 -> [w531]
        frame #0 {
          n248 = while {
            tunnel: [w523] -> w515
            tunnel: [w517] -> w514
            i -> [w516]
            stop <- w518 stop-if-true
            n249 = local read "cam receive port"() -> (w528:u16)
            n250 = local read "cam send port"() -> (w525:u16)
            n251 = call "UDPreceiver.vi"("sender's port"=w525, "receiver's port"=w528, "timeout ms (5000)"=100, "sender's IP"="master IP", "r-t"=TRUE) -> ("error"=w522:bool, "data out"=w530:string)  [unwired: 5 in]
            n252 = Not(x=w522) -> (.not. x?=w519:bool)
            n253 = Unflatten From String(type=cluster{"frames to record":i32, string} {"frames to record"=0, ""} ("output cluster"), binary string=w530) -> (value=w523:cluster{"frames to record":i32, string})  [unwired: 3 in, 2 out]
            n254 = local read "result"() -> (w520:bool)
            n255 = Compound Arithmetic op=OR(w520, "force stop") -> (w517:bool)
            n256 = Compound Arithmetic op=OR(w517, w519) -> (w518:bool)
            "UDP wait" <- w516
          }
        }
        frame #1 {
          n257 = case shown="False" w531 {
            tunnel: w532 -> [w533 _]
            frame False {
              w536 = TRUE ("record imgs")
              # "masterと独立\nに変わる"
              n258 = Unbundle(w533) -> ("frames to record"=w534:i32, w535:string)
              n259 = local write "frames to record"(w534) -> ()
              n260 = local write "folder name"(w535) -> ()
              n261 = local write "REC"(w536) -> ()
              n262 = global write "Global 1.vi" "rec ready"(w536) -> ()
            }
            frame True {
            }
          }
        }
      }
    }
  }
  n263 = case shown="True" w30 {
    tunnel: w29 -> [w540 w582]
    tunnel: w28 -> [w542 w581]
    tunnel: [w542 w580] -> w25
    tunnel: w27 -> [w539 w579]
    tunnel: w10 -> [w541 w566]
    tunnel: [w541 w573] -> w26
    tunnel: [w540 w578] -> w17
    tunnel: [w539 w577] -> w16
    tunnel: w9 -> [w538 w556]
    tunnel: [w538 w555] -> w7
    tunnel: [w537 w554] -> w6
    tunnel: w5 -> [w537 w553]
    frame False {
    }
    frame True {
      # "aqcuire frames and timestamps"
      n264 = local read "master(F)/slave(T)"() -> (w547:bool)
      n265 = while {
        tunnel: [w868] -> w570
        stop <- w866 stop-if-true
        n266 = local read "folder name"() -> (w868:string)
        n267 = local read "rec start"() -> (w867:bool)
        n268 = Or(x=w867, y="force 2") -> (x .or. y?=w866:bool)
      }
      n269 = global read "filepath global variable.vi" "img save folder (slave)"() -> (w546:path)
      n270 = global read "filepath global variable.vi" "img save folder"() -> (w545:path)
      n271 = Select(t=w546, s=w547, f=w545) -> (s? t:f=w544:path)
      n272 = Build Path(base path=w544, name or relative path=w570) -> (appended path=w572:path)
      n273 = Create Folder(path (use dialog)=w572) -> (created path=w552:path, error out=→"error out 2":errorcluster)  [unwired: 2 in, 1 out]
      n274 = case shown="False" w547 {
        tunnel: [w879 w884] -> w568
        tunnel: [w877 w883] -> w569
        tunnel: w552 -> [w870 w882]
        tunnel: [w872 _] -> w567
        tunnel: [w869 _] -> w558
        frame False {
          n275 = Build Path(base path=w870, name or relative path="img-ch1.bin" ("string")) -> (appended path=w879:path)
          n276 = Build Path(base path=w870, name or relative path="waveforms.pico" ("string")) -> (appended path=w878:path)
          n277 = Build Path(base path=w870, name or relative path="timestamp-ch1.csv" ("string")) -> (appended path=w877:path)
          n278 = Build Path(base path=w870, name or relative path="config" ("config filename")) -> (appended path=w869:path)
          n279 = Build Path(base path=w870, name or relative path="bf.jpg" ("string")) -> (appended path=w872:path)
          n280 = global write "Global 1.vi" ".pico filepath"(w878) -> ()
        }
        frame True {
          n281 = Build Path(base path=w882, name or relative path="timestamp-ch2.csv" ("string")) -> (appended path=w883:path)
          n282 = Build Path(base path=w882, name or relative path="img-ch2.bin" ("string")) -> (appended path=w884:path)
        }
      }
      n283 = Not(x=w547) -> (.not. x?=w548:bool)
      n284 = And(x=w548, y="save BF video") -> (x .and. y?=w549:bool)
      n285 = case shown="True" w549 {
        tunnel: w556 -> [w584 w591]
        tunnel: [w584 w590] -> w555
        tunnel: [w583 w589] -> w554
        tunnel: w553 -> [w583 w588]
        tunnel: w552 -> [w585 w587]
        tunnel: [w585 w586] -> w551
        frame False {
        }
        frame True {
          w592 = u32 5  # Num of Img Buffers
          n286 = for "For Loop_template0" {
            N: w592 -> [_]
            tunnel: [w629] -> w594 mode=indexing
            i -> [w628]
            n287 = Format Into String(format string="Basler rec %d" ("Image Name"), w628) -> (resulting string=w625:string)  [unwired: 2 in, 1 out]
            n288 = call "IMAQ Create"("Border Size"=3, "Image Name"=w625) -> ("New Image"=w629:T14)  [unwired: 2 in, 2 out]
          }
          n289 = call <vilib>:"IMAQdx Configure Acquisition.vi"("error in"=w588, "Number of Buffers"=w592, "Continuous?"=IMAQdx_Acquisition_Mode."Continuous", "Session In"=w591) -> ("error out"=w597:errorcluster, "Session Out"=w598:T8)  [unwired: 6 out]
          n290 = call <vilib>:"IMAQdx Start Acquisition.vi"("error in"=w597, "Session In"=w598) -> ("error out"=w593:errorcluster, "Session Out"=w595:T8)  [unwired: 8 out]
          n291 = while {
            tunnel: w594 -> [w620]
            tunnel: w593 -> [w607]
            tunnel: w595 -> [w606]
            tunnel: [w604] -> w589
            tunnel: [w603] -> w590
            tunnel: w587 -> [w601]
            tunnel: [w601] -> w586
            i -> [w608]
            stop <- w605 stop-if-true
            w619 = TRUE  # Log Image
            w618 = "Image"  # Image Logging Prefix
            # "record BF movie"
            n292 = Array Size(array=w620) -> (size(s)=w611:i32)
            n293 = Quotient & Remainder(x=w608, y=w611) -> (x-y*floor(x/y)=w612:i32)  [unwired: 1 out]
            n294 = Index Array(array=w620, index=w612) -> (element=w613:T14)
            n295 = call <vilib>:"IMAQdx Get Image2.vi"("Timeout (ms)"=-2, "Buffer Number Mode (Next)"=IMAQdx_Buffer_Number_Mode."Every", "error in"=w607, "Image In"=w613, "Session In"=w606) -> ("error out"=w610:errorcluster, "Image Out"=w624:T14, "Session Out"=w609:T8)  [unwired: 3 in, 1 out]
            n296 = property class="IMAQdx"(reference=w609, error in=w610) -> (reference out=w603:T8, error out=w614:errorcluster, "Status Information:Lost Buffer Count"=→"Lost Imgs":u32, "Status Information:Last Buffer Count"=→"Tot Img Trans":u32)
            n297 = local read "stop acq"() -> (w599:bool)
            n298 = Or(x="Stop (F)", y=w599) -> (x .or. y?=w600:bool)
            n299 = call <vilib>:"Vision Acquisition Image Logging.vi"("File Settings"=T19 {"File Type"="AVI", "Quality"=750, "Compress"=FALSE, "Lossless"=TRUE, "Ratio"=50.0, "Codec"="Motion JPEG (NI Vision)", "Frame Rate"=25, "Limit Frames"=FALSE, "Max Frames"=10} ("output cluster"), "Close"=w600, "Log Image"=w619, "error in (no error)"=w614, "Image Logging Prefix"=w618, "Image Logging Path"=w601, "Image In"=w624) -> ("error out"=w604:errorcluster)  [unwired: 4 out]
            n300 = Unbundle By Name(w604) -> ("status"=w617:bool)
            n301 = Or(x=w617, y=w600) -> (x .or. y?=w605:bool)
            "BF save idx" <- w608
          }
        }
      }
      n302 = Open/Create/Replace File(file path (use dialog)=w568, operation (0:open)=T17."open or create") -> (refnum out=w576:refnum<file>)  [unwired: 4 in, 2 out]
      n303 = local read "frames to record"() -> (w557:u32)
      n304 = while {
        tunnel: w582 -> [w905]
        tunnel: w581 -> [w904]
        tunnel: [w903] -> w580
        tunnel: w579 -> [w901]
        tunnel: w566 -> [w900]
        tunnel: [w899] -> w573
        tunnel: [w898] -> w578
        tunnel: [w897] -> w577
        tunnel: w576 -> [w896]
        tunnel: [w895] -> w575
        tunnel: w557 -> [w888]
        tunnel: [w886] -> w543 mode=indexing
        i -> [w892]
        stop <- w894 stop-if-true
        w902 = 10000 ("timeout in ms (-1)")
        n305 = Decrement(x=w888) -> (x-1=w890:u32)
        n306 = Dequeue Element(queue=w905, timeout in ms (-1)=w902, error in (no error)=w904) -> (queue out=w898:refnum<queue>, element=w887:u16[][], timed out?=w893:bool, error out=w903:errorcluster)
        n307 = Dequeue Element(queue=w901, timeout in ms (-1)=w902, error in (no error)=w900) -> (queue out=w897:refnum<queue>, element=w886:dbl, error out=w899:errorcluster)  [unwired: 1 out]
        n308 = Greater Or Equal?(x=w892, y=w890) -> (x >= y?=w891:bool)
        n309 = Or(x=w893, y=w891) -> (x .or. y?=w894:bool)
        "stop acq" <- w894
        n310 = case shown="True" TRUE {
          tunnel: w896 -> [w912 w915]
          tunnel: [w912 w914] -> w895
          tunnel: w887 -> [_ w913]
          frame False {
          }
          frame True {
            # "record imgs"
            n311 = Write to Binary File(file (use dialog)=w915, data=w913) -> (refnum out=w914:refnum<file>)  [unwired: 4 in, 2 out]
          }
        }
        n312 = case shown="True" "UDP send vol img" {
          tunnel: w887 -> [_ w911]
          tunnel: w886 -> [_ w906]
          frame False {
          }
          frame True {
            w910 = 65507  # Packet size
            # "send image frames by UDP"
            n313 = local read "img receive port"() -> (w907:u16)
            n314 = local read "img process IP"() -> (w908:string)
            n315 = local read "img send port"() -> (w909:u16)
            n316 = call "UDP volume send (subVI).vi"("timestamp"=w906, "Packet size"=w910, "local port"=w909, "port of receiver"=w907, "address"=w908, "frame data"=w911) -> ()  [unwired: 5 in, 1 out]
          }
        }
        "file index" <- w892
      }
      n317 = flat-sequence {
        tunnel: w567 -> [w632]
        tunnel: w568 -> [w633]
        tunnel: w569 -> [w634]
        tunnel: w551 -> [w635]
        tunnel: w575 -> [w636]
        tunnel: w543 -> [w637]
        tunnel: [w637] -> w565
        tunnel: [w636] -> w564
        tunnel: [w635] -> w563
        tunnel: [w634] -> w562
        tunnel: [w633] -> w561
        tunnel: [w632] -> w560
        tunnel: [w630] -> w559
        tunnel: w558 -> [w630]
        tunnel: w573 -> [w651]
        tunnel: w565 -> [w642]
        tunnel: w564 -> [w653]
        tunnel: w563 -> [w650]
        tunnel: w562 -> [w649]
        tunnel: w561 -> [w648]
        tunnel: w560 -> [w647]
        tunnel: w559 -> [w644]
        frame #0 {
          n318 = Wait (ms)(milliseconds to wait=u32 1000) -> ()  [unwired: 1 out]
        }
        frame #1 {
          w643 = TRUE  # newer than 240815
          n319 = Close File(refnum=w653) -> (error out=w646:errorcluster)  [unwired: 1 in, 1 out]
          n320 = call "diffrerential array.vi"("Array in"=w642) -> ("Array"=w641:dbl[])  [unwired: 10 in]
          "timestamp intervals" <- w641
          n321 = Delete From Array(array=w641, length=1) -> ()  [unwired: 1 in, 2 out]
          n322 = global read "global for picoscope.vi" "dead time for burst [us]"() -> (w657:dbl)
          n323 = global read "global for picoscope.vi" "AOD scan speed ratio"() -> (w666:dbl)
          n324 = global read "global for picoscope.vi" "g2 period [us]"() -> (w661:dbl)
          n325 = Multiply(x=1000000.0, y=w642) -> (x*y=w656:dbl[])
          n326 = global read "global for picoscope.vi" "Nzf"() -> (w664:i32)
          n327 = global read "global for picoscope.vi" "Nv"() -> (w662:i32)
          n328 = global read "global for picoscope.vi" "Nx"() -> (w663:dbl)
          n329 = case shown="True" w643 {
            tunnel: w656 -> [w669 w671]
            tunnel: [w668 w671] -> w655
            frame False {
              n330 = Delete From Array(array=w669, length=1 ("index")) -> (array with subset deleted=w668:dbl[])  [unwired: 1 in, 1 out]
            }
            frame True {
            }
          }
          n331 = local read "master(F)/slave(T)"() -> (w652:bool)
          n332 = Build Array(w662, w664, w663, w666, w661, w657) -> (w659:dbl[])
          n333 = local read "one PC"() -> (w640:bool)
          n334 = Insert Into Array(array=w655, index=0, new element=w659) -> (w658:dbl[])
          n335 = Not(x=w640) -> (.not. x?=w638:bool)
          n336 = call-poly <vilib>:"Write Delimited Spreadsheet.vi"("file path (dialog if empty)"=w649, "format (%.3f)"="%.8f", "1D data"=w658) -> ("error out"=w645:errorcluster)  [unwired: 11 in, 1 out]
          n337 = And(x=w638, y=w652) -> (x .and. y?=w639:bool)
          n338 = case shown="False" w639 {
            tunnel: w650 -> [w676 _]
            tunnel: w651 -> [_ w859]
            tunnel: w649 -> [_ w853]
            tunnel: w648 -> [_ w854]
            tunnel: w647 -> [w705 _]
            tunnel: w646 -> [_ _]
            tunnel: w645 -> [w688 _]
            tunnel: w644 -> [w700 _]
            tunnel: w642 -> [w689 _]
            frame False {
              # "開いているアプリの中から顕微鏡システム制御用VI(scape image acquisitionxxx.vi)を探して制御器の値をすべて保存"
              n339 = local read "time ofst"() -> (w690:dbl)
              n340 = global read "filepath global variable.vi" "save_time.txt"() -> (w692:path)
              n341 = call "create timestamp text file (seconds for HHMMSS.SSS)(SubVI).vi"("error in"=w688, "time offset"=w690, "Array"=w689, "appended path"=w692) -> ("error out"=w686:errorcluster)  [unwired: 7 in]
              n342 = global read "filepath global variable.vi" "masterPC filesave"() -> (w694:path)
              n343 = local read "folder name"() -> (w687:string)
              n344 = Build Path(base path=w694, name or relative path=w687) -> (appended path=w693:path)
              n345 = Path To String(path=w693) -> (string=w695:string)
              n346 = global read "filepath global variable.vi" "save_path.txt"() -> (w691:path)
              n347 = Write to Text File(file (use dialog)=w691, text=w695, error in=w686) -> (error out=w685:errorcluster)  [unwired: 1 in, 2 out]
              n348 = local read "slice cut pos"() -> (w704:path)
              n349 = call "use designated z spacing (SubVI).vi"("use designated z spacing"=FALSE, "file path"=w704) -> ("path"=w703:path)  [unwired: 1 in]
              n350 = Copy(8:w685, 9:TRUE ("overwrite (F)"), 10:w676, 11:w703) -> (0:w684:errorcluster)  [unwired: 1 in, 2 out]
              n351 = case shown="True" TRUE {
                tunnel: w705 -> [_ w846]
                tunnel: w684 -> [w843 w845]
                tunnel: [w843 w844] -> w683
                frame False {
                }
                frame True {
                  n352 = invoke on="BF" class="Pict" method="Get Image"("image depth"=24 ("Image Depth"), "bg color"=u32 0 ("Background Color")) -> ("image data"=w847:T21)  [unwired: 4 in, 5 out]
                  n353 = call <vilib>:"Write JPEG File.vi"("error in (no error)"=w845, "image data"=w847, "path to JPEG file"=w846) -> ("error out"=w844:errorcluster)  [unwired: 7 in, 1 out]
                }
              }
              n354 = property class="App"() -> ("App.AllVIsPaths"=w699:string[])  [unwired: 2 in, 2 out]
              n355 = for {
                tunnel: w699 -> [w722] mode=indexing
                tunnel: [w722] -> w698 if=w721
                n356 = xnode "Match Regular Expression"("input string"=w722, "regular expression"="scape image aqcuisition") -> ("whole match"=w724:string)  [unwired: 4 in, 4 out]
                n357 = String Length(string=w724) -> (length=w723:i32)
                n358 = Greater Than 0?(x=w723) -> (x > 0?=w721:bool)
              }
              n359 = String To Path(string=w698) -> (path=w697:path)
              n360 = Open VI Reference(vi path=w697) -> (vi reference=w696:refnum<vi>)  [unwired: 5 in, 1 out]
              n361 = call "SaveControlValues.vi"("Mode"=enum16{"Save", "Load"}."Save" ("Save Control Values Mode"), "エラー入力"=w683, "file path"=w700, "Target VI"=w696) -> ("error out"=w675:errorcluster)  [unwired: 1 in, 6 out]
              n362 = case shown="True" "use most recent 2" {
                tunnel: "folder for imgcalib.txt" -> [w713 w719]
                tunnel: [w713 w715] -> w672
                frame False {
                }
                frame True {
                  n363 = Strip Path(path=w719) -> (stripped path=w720:path)  [unwired: 1 out]
                  n364 = call "Find The Most File 2012 NIVerified.vi"("pattern"="*-cropbulkcalib", "file(T)/folder(F)"=FALSE, "Folder Path In"=w720) -> ("File Path Out"=w714:path)  [unwired: 7 in, 1 out]
                  n365 = local write "folder for imgcalib.txt"(w714) -> ()
                  n366 = Build Path(base path=w714, name or relative path="imgcalib.txt") -> (appended path=w715:path)
                }
              }
              n367 = Not Equal?(x=w672, y=path "" ("source path 3")) -> (x != y?=w680:bool)
              n368 = call <vilib>:"Check if File or Folder Exists.vi"("path"=w672) -> ("file or folder exists?"=w681:bool)  [unwired: 8 in, 2 out]
              n369 = And(x=w680, y=w681) -> (x .and. y?=w673:bool)
              n370 = case shown="True" w673 {
                tunnel: w676 -> [_ w712]
                tunnel: w672 -> [_ w710]
                tunnel: w675 -> [w707 w709]
                tunnel: [w707 w708] -> w674
                frame False {
                }
                frame True {
                  n371 = Copy(8:w709, 9:TRUE ("overwrite (F)"), 10:w712, 11:w710) -> (0:w708:errorcluster)  [unwired: 1 in, 2 out]
                }
              }
              "error out 3" <- w674
            }
            frame True {
              # "2ch記録の場合はslave PCからファイルをコピーする"
              n372 = global read "filepath global variable.vi" "masterPC filesave"() -> (w851:path)
              n373 = local read "folder name"() -> (w856:string)
              n374 = Strip Path(path=w853) -> (name=w852:string)  [unwired: 1 out]
              n375 = Build Path(base path=w851, name or relative path=w856) -> (appended path=w855:path)
              n376 = Build Path(base path=w855, name or relative path=w852) -> (appended path=w857:path)
              n377 = Move(source path=w853, error in=w859, 10:w857) -> (error out=w858:errorcluster)  [unwired: 2 in, 2 out]
              n378 = case shown="False" "copy later" {
                tunnel: w858 -> [w864 _]
                tunnel: w855 -> [w862 _]
                tunnel: w854 -> [w861 _]
                frame False {
                  n379 = Strip Path(path=w861) -> (name=w860:string)  [unwired: 1 out]
                  n380 = Build Path(base path=w862, name or relative path=w860) -> (appended path=w863:path)
                  n381 = Move(source path=w861, error in=w864, 10:w863) -> ()  [unwired: 2 in, 3 out]
                }
                frame True {
                }
              }
            }
          }
        }
      }
    }
  }
  n382 = local read "master(F)/slave(T)"() -> (w12:bool)
  n383 = Release Queue(queue=w17, error in (no error)=w25) -> (error out=w22:errorcluster)  [unwired: 1 in, 2 out]
  n384 = call <vilib>:"IMAQdx Close Camera.vi"("error in"=w6, "Session In"=w7) -> ("error out"=→"error out 4":errorcluster)  [unwired: 9 out]
  n385 = Release Queue(queue=w16, error in (no error)=w26) -> ()  [unwired: 1 in, 3 out]
  n386 = case shown="False" w12 {
    tunnel: w14 -> [w916 _]
    tunnel: w13 -> [w918 _]
    frame False {
      n387 = call "IMAQ Dispose"("Image"=w916, "error in (no error)"=w918) -> ("error out"=→"Error Out":errorcluster)  [unwired: 4 in]
    }
    frame True {
    }
  }
  n388 = flat-sequence {
    tunnel: w22 -> [_]
    tunnel: w15 -> [_]
    frame #0 {
      w919 = TRUE ("receive")
      w920 = FALSE ("receive")
      n389 = global write "Global 1.vi" "record"(w920) -> ()
      n390 = global write "Global 1.vi" "rec ready 2"(w920) -> ()
      n391 = local write "result"(w920) -> ()
      n392 = global write "Global 1.vi" "rec stop [Cam->Pico]"(w920) -> ()
      n393 = local write "calib"(w920) -> ()
      n394 = global write "Global 1.vi" "calib"(w920) -> ()
      n395 = global write "Global 1.vi" "rec ready"(w920) -> ()
      n396 = local write "rec ready"(w920) -> ()
      n397 = local write "REC"(w920) -> ()
      n398 = property on="one PC" class="Bool (strict)"("Visible"=w919) -> ()  [unwired: 2 in, 2 out]
      n399 = property on="BF" class="Pict"("Visible"=w919) -> ()  [unwired: 2 in, 2 out]
      n400 = property on="copy later" class="Bool (strict)"("Visible"=w919) -> ()  [unwired: 2 in, 2 out]
      n401 = property on="control picoscope dependent enable" class="Bool (strict)"("Visible"=w919) -> ()  [unwired: 2 in, 2 out]
      n402 = property on="calib" class="Bool (strict)"("Visible"=w919) -> ()  [unwired: 2 in, 2 out]
      n403 = property on="REC" class="Bool (strict)"("Visible"=w919) -> ()  [unwired: 2 in, 2 out]
    }
  }
  "sCMOS" <- FALSE
